vi "AnalogDisc_Core.vi"(8 "error in":errorcluster, 9 "SignalBufferQueue in":refnum<queue>, 10 "DWFCtrlQueue in":refnum<queue>, 11 "DevSN":string="210244449465") -> (0 "error out":errorcluster)   [LabVIEW 2013, in "AnalogDiscSDKLv.lvlib"]
uses:
  <instrlib>/AnalogDiscSDKLv/AnalogDiscSDKLv.lvlib
  <instrlib>/AnalogDiscSDKLv/VIs/DWF_AnalogIn_Configurations.ctl
  <instrlib>/AnalogDiscSDKLv/VIs/DWF_AcqMode.ctl
  <instrlib>/AnalogDiscSDKLv/VIs/DWF_Filter.ctl
  <instrlib>/AnalogDiscSDKLv/VIs/DWF_TrigSrc.ctl
  <instrlib>/AnalogDiscSDKLv/VIs/DWF_TrigCond.ctl
  <instrlib>/AnalogDiscSDKLv/VIs/DWF_TrigType.ctl
  <instrlib>/AnalogDiscSDKLv/VIs/DWF_CtrlQueue.ctl
  <instrlib>/AnalogDiscSDKLv/VIs/DWF_State.ctl
  <instrlib>/AnalogDiscSDKLv/VIs/DWF_PrivateStats.ctl
  <instrlib>/AnalogDiscSDKLv/VIs/DWF_InstrumentStatus.ctl
  <instrlib>/AnalogDiscSDKLv/VIs/DWF_DwfState.ctl
  <instrlib>/AnalogDiscSDKLv/VIs/DWF_Signal.ctl
  <instrlib>/AnalogDiscSDKLv/VIs/DWF_TrigLen.ctl
  <instrlib>/AnalogDiscSDKLv/VIs/DWF_DWFERC.ctl
  <vilib>/Utility/error.llb/DialogType.ctl
  <instrlib>/AnalogDiscSDKLv/VIs/DWF_AnalogOut_ChannelConfigurations.ctl
  <instrlib>/AnalogDiscSDKLv/VIs/DWF_Function.ctl
  <instrlib>/AnalogDiscSDKLv/VIs/DWF_Node.ctl
  <vilib>/Utility/miscctls.llb/LVPositionTypeDef.ctl
  <vilib>/Analysis/1siggen.llb/Ramp Pattern by Samples.vi
  <vilib>/Utility/error.llb/Error Cluster From Error Code.vi
  <vilib>/ErrorRing/Error Ring.xnode
  <vilib>/ptbypt/NI_PtbyPt.lvlib
  <userlib>/Utility/ErrorLog_lib.lvlib
  C:/Windows/System32/dwf.dll
  <vilib>/Analysis/NI_AALBase.lvlib
panel:
  out "WaitForVoltageStablize":bool
  in  "GetInfo":bool
  out "psecPosition":dbl
  out "elements":T1[](array[typedef])
  out "sysCount_inPCTrig":i32
  out "PCTrig_counter":i32
  out "AO2_sts":T3=enum."Armed"
  out "AO1_sts":T3=enum."Armed"
  in  "fStart_AO":bool
  in  "SetFuncData_AO":bool
  in  "SetTrigSrc_AO":bool
  in  "SetEnable_AO":bool
  in  "SetConfig_AO":bool
  in  "SetStates_AO":bool
  out "waited t PCTrig":u32
  out "AI_sts":T4
  in  "TriggerPC":bool
  out "Live Stats":T5
  in  "Mode(N/T)":bool caption="Mode"
  out "Graph":sgl[][](graph)
  in  "fConfig":bool
  in  "Reset":bool
  in  "CloseAll":bool
  in  "Close":bool
  in  "Enumerate":bool
  in  "Open":bool
  in  "Quit":bool
  in  "Start":bool
  in  "ConfigAll":bool
  out "UserName":string[](array[string])
  out "SN":string[](array[string])
  out "DevName":string[](array[string])
  out "DeviceID":i32[](array[numeric])
  out "pnDevice":i32
  out "isBusy":i32[](array[numeric])
  out "DeviceVersion":i32[](array[numeric])
  in  "Configurations":T6={"Acqusition"={"Freq(Hz,SampleRate)"=10000000.0, "BufferSize"=8192, "Mode"=enum."Single", "RecordLength(s)"=0.0008192}, "Channels"=[{"Range(V)"=5.0, "Offset(V)"=0.0, "Filter"=enum."Decimate", "Enable"=TRUE}], "Trigger"={"TriggerSource"=enum."None", "Timeout(s)"=0.0, "Holdoff(s)"=1e-06, "Position/Delay(s)"=0.0}, "AnalogTrigger"={"Channel"=0, "Polarity"=enum."Rising", "Type"=enum."Pulse", "Level(V)"=0.0, "Filter"=enum."MinMax", "Hysterisis(V)"=0.0}} {"AnalogTrigger"."Channel" format="%#_6p"; "AnalogTrigger"."Hysterisis(V)" format="%#_6p"; "Acqusition"."RecordLength(s)" format="%#_6p"; "Acqusition"."Freq(Hz,SampleRate)" format="%#_6p"; "Acqusition"."BufferSize" min=1 max=16384 step=1; "Trigger"."Position/Delay(s)" format="%#_6p"; "Trigger"."Holdoff(s)" format="%#_6p"}
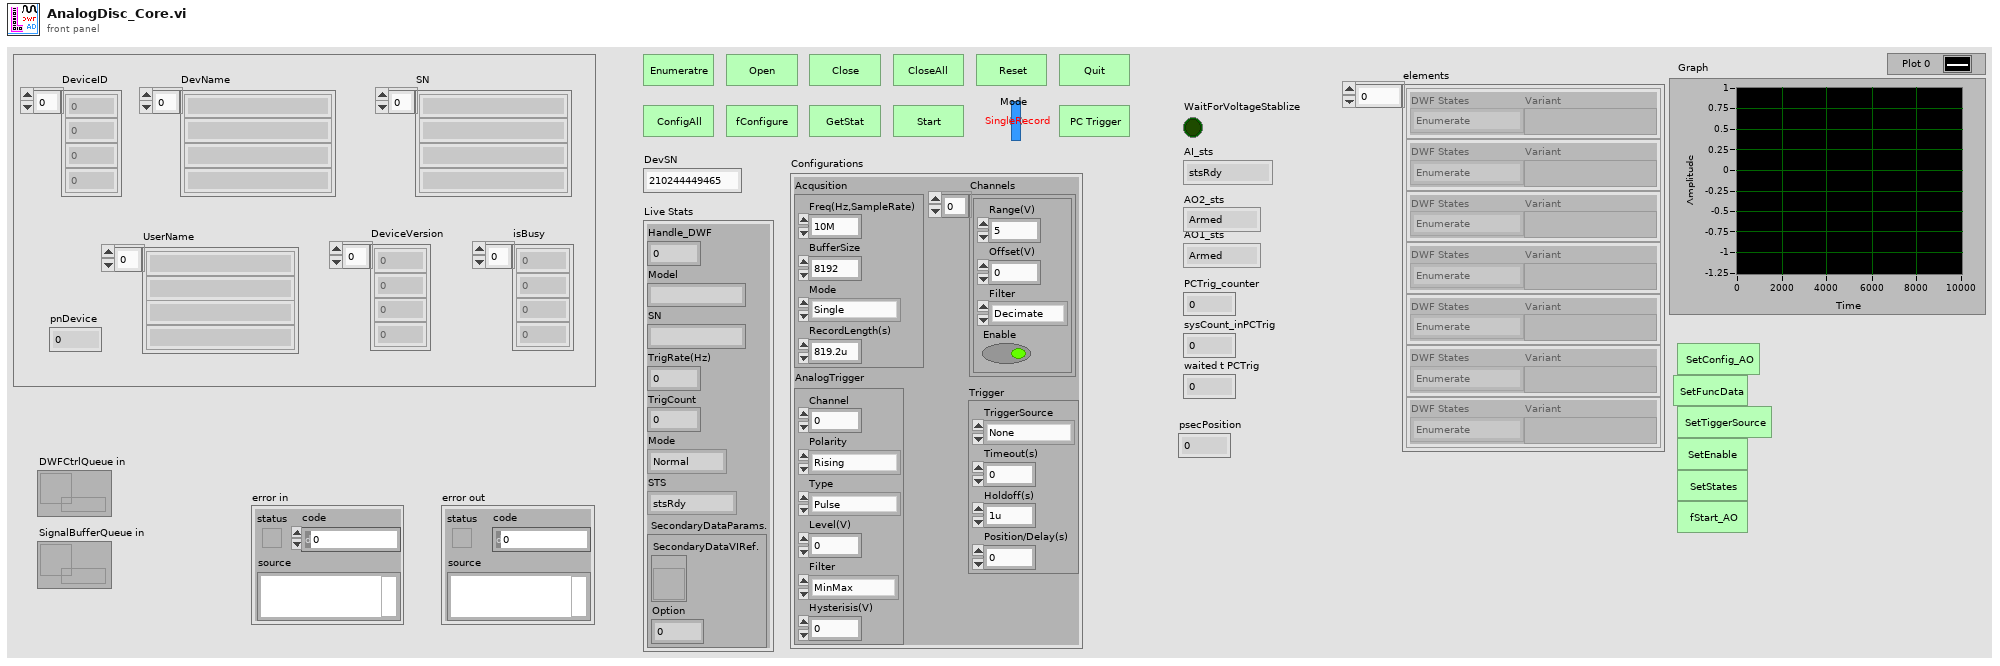
[diagram p1: front panel]
types:
  T1 = typedef "AnalogDiscSDKLv.lvlib/DWF_CtrlQueue.ctl" = cluster{"DWF States":T2, "Variant":variant}
  T2 = typedef "AnalogDiscSDKLv.lvlib/DWF_State.ctl" = enum16{"Enumerate", "Open", "Close", "CloseAll", "Reset", "Quit", "==Settings==", "SetAcquisition_", "SetChannels_", "SetTrigger_", "SetAnalogTrigDetector_", "SetAll_AcquChTrig_", "fConfigurate", "fStart", "GetStatus", "_WaitForDone/Idle", "_GetData", "GetAcquisition", "GetChannels", "GetTrigger", "GetAll_AcquChTrig", "==Messaging==", "_PushDataOut", "GetStat_", "GetConfig_", "==ModeSetup==", "SetSignalBuffer_", "SetMode_", "SetSecondaryDataRef._", "==AnalogOut==", "GetChannelCount_AO", "fStart_AO", "SetChEnable_AO", "SetConfig_AO", "SetFuncData_AO", "SetOffset_AO_", "SetMasterNode_AO", "SetStates_AO", "SetSymetry_AO", "SetTriggerSource_AO", "==Trigger==", "ManualTrigger"}
  T3 = typedef "AnalogDiscSDKLv.lvlib/DWF_DwfState.ctl" = enum16{"Ready", "Armed", "Done", "Running", "Config", "Prefill", "---", "Wait"}
  T4 = typedef "AnalogDiscSDKLv.lvlib/DWF_InstrumentStatus.ctl" = enum16{"stsRdy", "stsARM", "stsDone", "stsTrig", "stsCfg", "stsPrefill", "stsNotDone", "stsTrigDly", "stsError", "stsBusy", "stsStop"}
  T5 = typedef "AnalogDiscSDKLv.lvlib/DWF_PrivateStats.ctl" = cluster{"Handle_DWF":i32, "Model":string, "SN":string, "TrigRate(Hz)":dbl, "TrigCount":i32, "Mode":enum16{"Normal", "Turbo"}, "STS":T4, "SecondaryDataParams.":cluster{"SecondaryDataVIRef.":refnum<vi>, "Option":i32}}
  T6 = typedef "AnalogDiscSDKLv.lvlib/DWF_AnalogIn_Configurations.ctl" = cluster{"Acqusition":cluster{"Freq(Hz,SampleRate)":dbl, "BufferSize":i32, "Mode":T7, "RecordLength(s)":dbl}, "Channels":cluster{"Range(V)":dbl, "Offset(V)":dbl, "Filter":T8, "Enable":bool}[], "Trigger":cluster{"TriggerSource":T9, "Timeout(s)":dbl, "Holdoff(s)":dbl, "Position/Delay(s)":dbl}, "AnalogTrigger":cluster{"Channel":i32, "Polarity":T10, "Type":T11, "Level(V)":dbl, "Filter":T8, "Hysterisis(V)":dbl}}
  T7 = typedef "AnalogDiscSDKLv.lvlib/DWF_AcqMode.ctl" = enum16{"Single", "ScanShift", "ScanScreen", "Record"}
  T8 = typedef "AnalogDiscSDKLv.lvlib/DWF_Filter.ctl" = enum16{"Decimate", "Average", "MinMax"}
  T9 = typedef "AnalogDiscSDKLv.lvlib/DWF_TrigSrc.ctl" = enum16{"None", "PC", "DetectorAnalogIn", "DetectorDigitalIn", "AnalogIn", "DigitalIn", "DigitalOut", "AnalogOut1", "AnalogOut2", "AnalogOut3", "AnalogOut4", "External1", "External2", "External3", "External4"}
  T10 = typedef "AnalogDiscSDKLv.lvlib/DWF_TrigCond.ctl" = enum16{"Rising", "Falling"}
  T11 = typedef "AnalogDiscSDKLv.lvlib/DWF_TrigType.ctl" = enum16{"Edge", "Pulse", "Transition"}
  T12 = typedef "LVPositionTypeDef.ctl" = cluster{"Left":i32, "Top":i32}
  T13 = typedef "AnalogDiscSDKLv.lvlib/DWF_AnalogOut_ChannelConfigurations.ctl" = cluster{"FUNC":T14, "Frequency(Hz)_AO":dbl, "Amplitude(V)_AO":dbl, "Phase(deg)_AO":dbl, "Offset(V)_AO":dbl, "rgdData":dbl[], "cData":i32, "Symmetry":dbl, "Enable":bool, "Node":T15}
  T14 = typedef "AnalogDiscSDKLv.lvlib/DWF_Function.ctl" = u8
  T15 = typedef "AnalogDiscSDKLv.lvlib/DWF_Node.ctl" = enum16{"Carrier", "FM", "AM"}
  T16 = cluster{"Configs":T13[], "ChannelCount":i32, "States":cluster{"Wait(s)":dbl, "Run(s)":dbl, "cRepeat":i32, "TriggerSource":T9}[]}
  T17 = typedef "DialogType.ctl" = u16
  T18 = typedef "AnalogDiscSDKLv.lvlib/DWF_DWFERC.ctl" = enum16{"dwfercNoErc", "dwfercUnknownError", "dwfercApiLockTimeout", "dwfercAlreadyOpened", "dwfercNotSupported", "dwfercInvalidParameter0", "dwfercInvalidParameter1", "dwfercInvalidParameter2", "dwfercInvalidParameter3"}
  T19 = typedef "AnalogDiscSDKLv.lvlib/DWF_TrigLen.ctl" = enum16{"triglenLess", "triglenTimeout", "triglenMore"}
  T20 = typedef "AnalogDiscSDKLv.lvlib/DWF_Signal.ctl" = cluster{"tickcount":u32, "Signal":sgl[][], "SecondaryData":dbl[]}
  T21 = cluster{"Freq(Hz,SampleRate)":dbl, "BufferSize":i32, "Mode":T7, "RecordLength(s)":dbl}
  T22 = cluster{"Range(V)":dbl, "Offset(V)":dbl, "Filter":T8, "Enable":bool}[]
  T23 = cluster{"TriggerSource":T9, "Timeout(s)":dbl, "Holdoff(s)":dbl, "Position/Delay(s)":dbl}
  T24 = cluster{"Channel":i32, "Polarity":T10, "Type":T11, "Level(V)":dbl, "Filter":T8, "Hysterisis(V)":dbl}
  T25 = cluster{"SecondaryDataVIRef.":refnum<vi>, "Option":i32}
  T26 = cluster{"Wait(s)":dbl, "Run(s)":dbl, "cRepeat":i32, "TriggerSource":T9}[]
  T27 = cluster{"Wait(s)":dbl, "Run(s)":dbl, "cRepeat":i32, "TriggerSource":T9}
  T28 = cluster{i32, "States":cluster{"Wait(s)":dbl, "Run(s)":dbl, "cRepeat":i32, "TriggerSource":T9}}
  T29 = typedef "DWF_AnalogIn_Configurations.ctl" = cluster{"Acqusition":cluster{"Freq(Hz,SampleRate)":dbl, "BufferSize":i32, "Mode":T30, "RecordLength(s)":dbl}, "Channels":cluster{"Range(V)":dbl, "Offset(V)":dbl, "Filter":T31, "Enable":bool}[], "Trigger":cluster{"TriggerSource":T32, "Timeout(s)":dbl, "Holdoff(s)":dbl, "Position/Delay(s)":dbl}, "AnalogTrigger":cluster{"Channel":i32, "Polarity":T33, "Type":T34, "Level(V)":dbl, "Filter":T31, "Hysterisis(V)":dbl}}
  T30 = typedef "DWF_AcqMode.ctl" = enum16{"Single", "ScanShift", "ScanScreen", "Record"}
  T31 = typedef "DWF_Filter.ctl" = enum16{"Decimate", "Average", "MinMax"}
  T32 = typedef "DWF_TrigSrc.ctl" = enum16{"None", "PC", "DetectorAnalogIn", "DetectorDigitalIn", "AnalogIn", "DigitalIn", "DigitalOut", "AnalogOut1", "AnalogOut2", "AnalogOut3", "AnalogOut4", "External1", "External2", "External3", "External4"}
  T33 = typedef "DWF_TrigCond.ctl" = enum16{"Rising", "Falling"}
  T34 = typedef "DWF_TrigType.ctl" = enum16{"Edge", "Pulse", "Transition"}
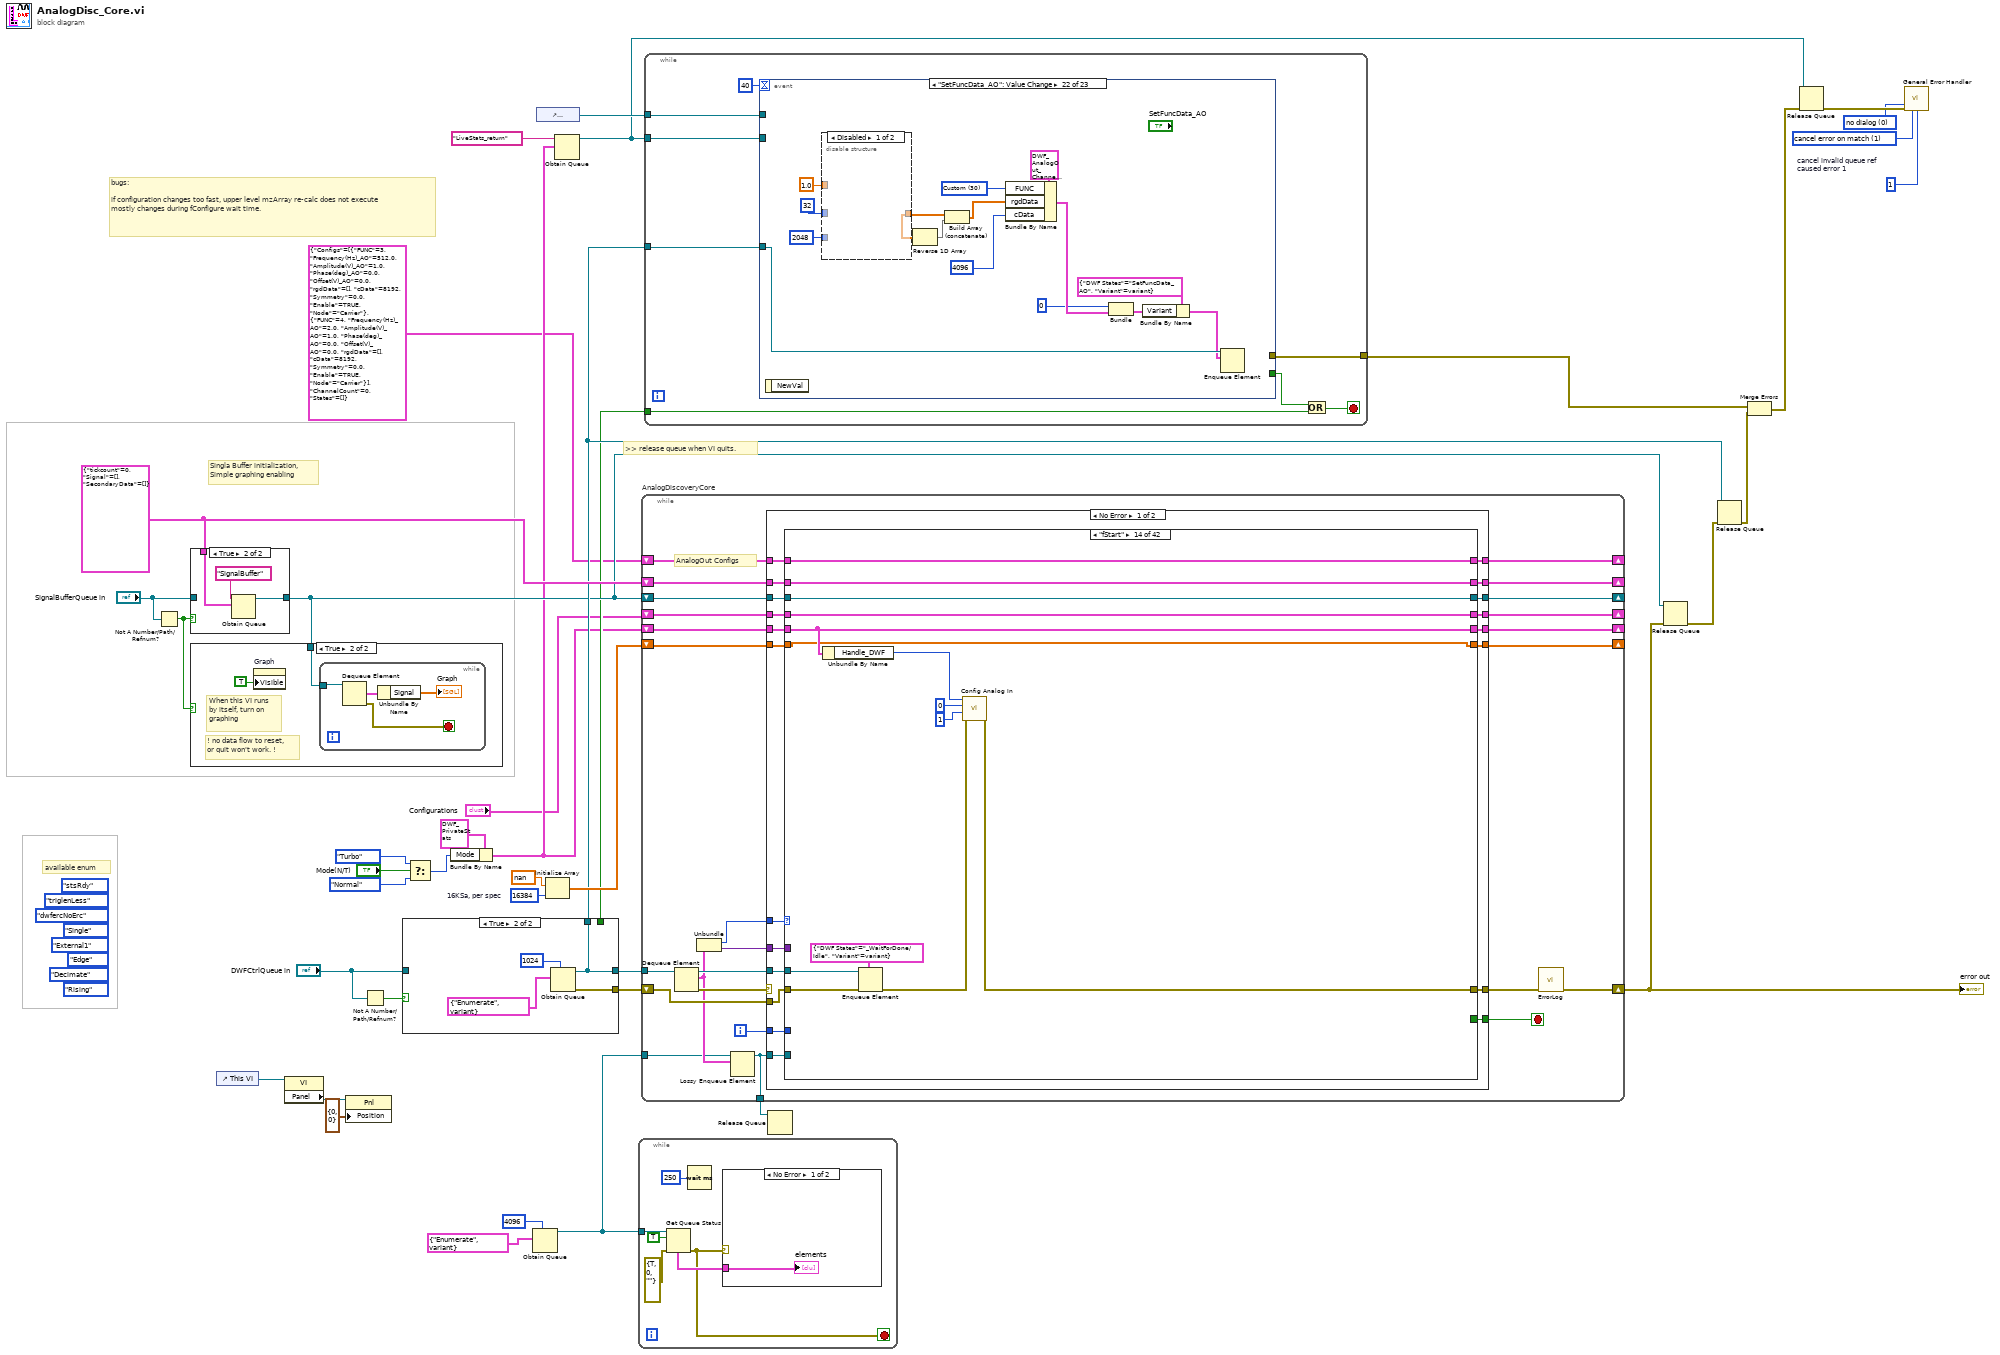
[diagram p0: block diagram]
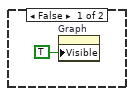
[diagram p3: hidden frame]
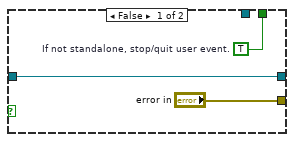
[diagram p5: hidden frame]
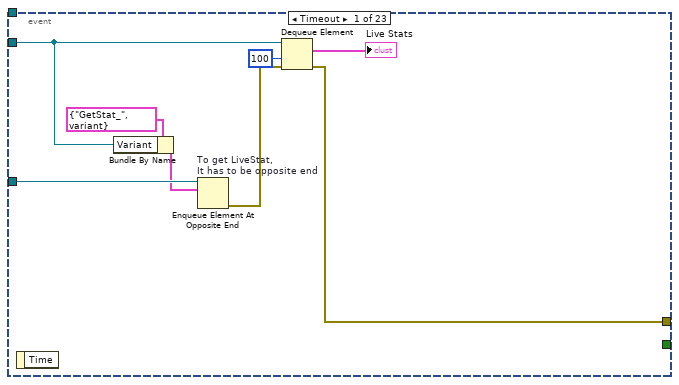
[diagram p6: hidden frame]
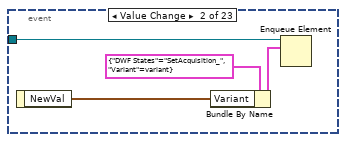
[diagram p7: hidden frame]
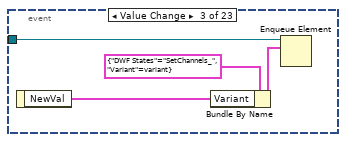
[diagram p8: hidden frame]
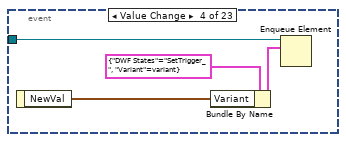
[diagram p9: hidden frame]
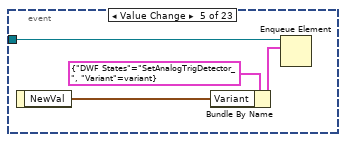
[diagram p10: hidden frame]
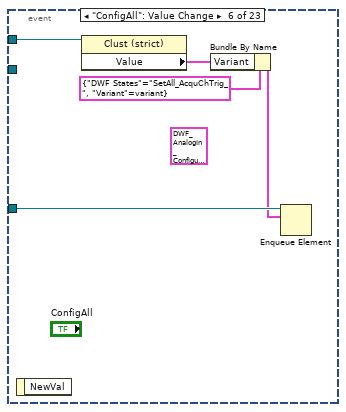
[diagram p11: hidden frame]
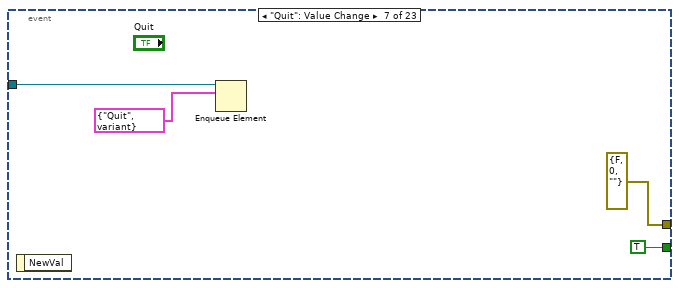
[diagram p12: hidden frame]
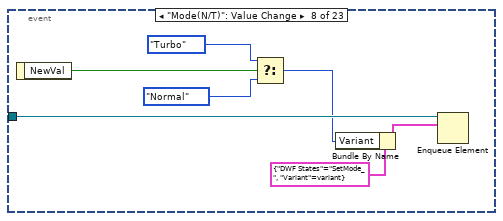
[diagram p13: hidden frame]
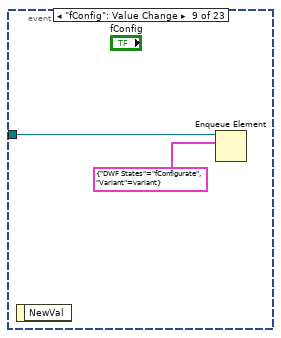
[diagram p14: hidden frame]
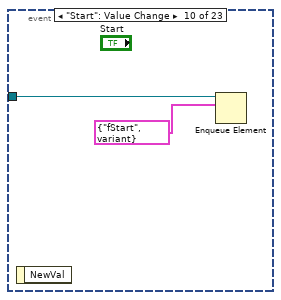
[diagram p15: hidden frame]
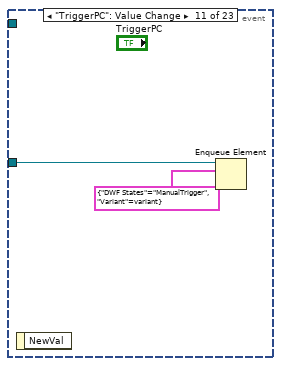
[diagram p16: hidden frame]
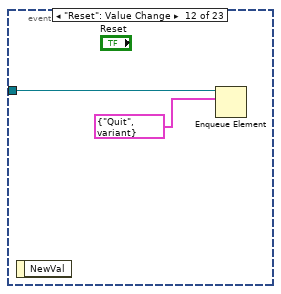
[diagram p17: hidden frame]
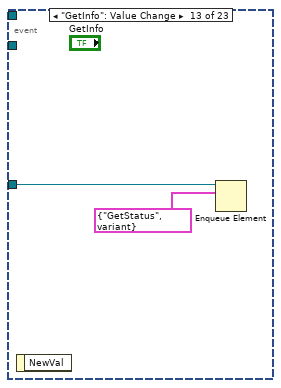
[diagram p18: hidden frame]
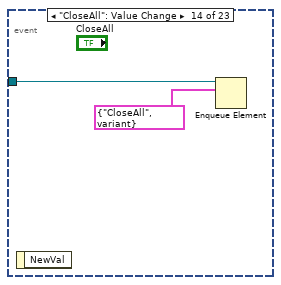
[diagram p19: hidden frame]
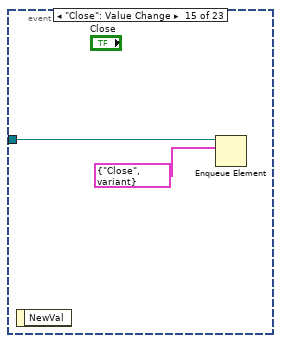
[diagram p20: hidden frame]
diagram:
  w19 = 1  # cancel invalid queue ref caused error 1
  w20 = 1 items=["no exception", "cancel error on match", "set error on match"] ("[exception action] (none:0)")
  w21 = T17 0 items=["no dialog", "OK message", "continue or stop message", "OK message + warnings", "continue/stop + warnings"] ("type of dialog (OK msg:1)")
  (unwired) DWF_TrigSrc."External1" ("TriggerSource")
  (unwired) DWF_DWFERC."dwfercNoErc" ("DWFErC")
  (unwired) DWF_TrigLen."triglenLess" ("TrigLen")
  (unwired) DWF_TrigCond."Rising" ("TrigCond")
  (unwired) DWF_TrigType."Edge" ("TrigType")
  (unwired) DWF_Filter."Decimate" ("Filter")
  (unwired) DWF_AcqMode."Single" ("ACQMODE")
  (unwired) DWF_InstrumentStatus."stsRdy" ("STS")
  w38 = 16384  # 16KSa, per spec
  w40 = T20 {"tickcount"=0, "Signal"=[], "SecondaryData"=[]} ("Signal_Typedef")
  # "bugs:\n\nif configuration changes too fast, upper level mzArray re-calc does not execute\nmostly changes during fConfigure wait time."
  # "Singla Buffer initialization,\nSimple graphing enabling"
  # "available enum"
  # ">> release queue when VI quits."
  n1 = Not A Number/Path/Refnum?(number/path/refnum="SignalBufferQueue in") -> (NaN/Path/Refnum?=w24:bool)
  n2 = case shown="True" w24 {
    tunnel: w40 -> [_ w44]
    tunnel: [w41 w43] -> w25
    tunnel: "SignalBufferQueue in" -> [w41 _]
    frame False {
    }
    frame True {
      n3 = Obtain Queue(name (unnamed)="SignalBuffer", element data type=w44) -> (queue out=w43:refnum<queue>)  [unwired: 3 in, 2 out]
    }
  }
  n4 = case shown="True" w24 {
    tunnel: w25 -> [_ w47]
    frame False {
      n5 = property on="Graph" class="WFGraph (strict)"("Visible"=TRUE) -> ()  [unwired: 2 in, 2 out]
    }
    frame True {
      # "! no data flow to reset,\nor quit won't work. !"
      # "When this VI runs\nby itself, turn on \ngraphing"
      n6 = property on="Graph" class="WFGraph (strict)"("Visible"=TRUE) -> ()  [unwired: 2 in, 2 out]
      n7 = while {
        tunnel: w47 -> [w51]
        stop <- w48 stop-if-true
        n8 = Dequeue Element(queue=w51) -> (element=w50:T20, error out=w48:errorcluster)  [unwired: 2 in, 2 out]
        n9 = Unbundle By Name(w50) -> ("Signal"=→"Graph":sgl[][])
      }
    }
  }
  n10 = control-ref of="This VI"() -> (w3:refnum<vi>)
  n11 = property class="VI"(reference=w3) -> ("Panel"=w2:refnum<vi>)  [unwired: 1 in, 2 out]
  n12 = property class="Pnl"(reference=w2, "Position"=T12 {"Left"=0, "Top"=0}) -> ()  [unwired: 1 in, 2 out]
  n13 = Not A Number/Path/Refnum?(number/path/refnum="DWFCtrlQueue in") -> (NaN/Path/Refnum?=w34:bool)
  n14 = case shown="True" w34 {
    tunnel: [w54 w55] -> w36
    tunnel: ["error in" w58] -> w35
    tunnel: "DWFCtrlQueue in" -> [w54 _]
    tunnel: [_ w55] -> w30
    tunnel: [w52 _] -> w18
    frame False {
      w52 = TRUE  # If not standalone, stop/quit user event.
    }
    frame True {
      n15 = Obtain Queue(max queue size (-1, unlimited)=1024, element data type=T1 {"DWF States"=enum."Enumerate", "Variant"=variant}) -> (queue out=w55:refnum<queue>, error out=w58:errorcluster)  [unwired: 3 in, 1 out]
    }
  }
  n16 = Select(t=enum16{"Normal", "Turbo"}."Turbo" ("Mode"), s="Mode(N/T)", f=enum16{"Normal", "Turbo"}."Normal" ("Mode")) -> (s? t:f=w11:enum16{"Normal", "Turbo"})
  n17 = Bundle By Name(cluster=T5 {"Handle_DWF"=0, "Model"="", "SN"="", "TrigRate(Hz)"=0.0, "TrigCount"=0, "Mode"=enum."Normal", "STS"=enum."stsRdy", "SecondaryDataParams."={"SecondaryDataVIRef."=refnum, "Option"=0}} ("PrivateStats(Live)"), "Mode"=w11) -> (w15:T5)
  n18 = Obtain Queue(max queue size (-1, unlimited)=4096, element data type=T1 {"DWF States"=enum."Enumerate", "Variant"=variant}) -> (queue out=w5:refnum<queue>)  [unwired: 3 in, 2 out]
  n19 = control-ref of="Configurations"() -> (w32:refnum<vi>)
  n20 = Initialize Array(nan ("Numeric"), w38) -> (w37:dbl[])
  n21 = Obtain Queue(name (unnamed)="LiveStats_return", element data type=w15) -> (queue out=w28:refnum<queue>)  [unwired: 3 in, 2 out]
  n22 = while {
    tunnel: w5 -> [w64]
    stop <- w61 stop-if-true
    n23 = Get Queue Status(queue=w64, return elements? (F)=TRUE, error in (no error)=errorcluster {"status"=TRUE, "code"=0, "source"=""}) -> (error out=w61:errorcluster, elements=w62:T1[])  [unwired: 6 out]
    n24 = Wait (ms)(milliseconds to wait=u32 250) -> ()  [unwired: 1 out]
    n25 = case shown="No Error" w61 {
      tunnel: w62 -> [w65 _]
      frame No Error {
        "elements" <- w65
      }
      frame Error {
      }
    }
  }
  n26 = while "AnalogDiscoveryCore" {
    shift-right: [w89] -> _
    shift-left: w25 -> [w90]
    tunnel: w36 -> [w71]
    shift-right: [w70] -> w23
    shift-left: w35 -> [w77]
    shift-right: [w86] -> _
    shift-left: "Configurations" -> [w85]
    shift-right: [w78] -> _
    shift-left: w15 -> [w84]
    shift-right: [w79] -> _
    shift-left: w37 -> [w82]
    shift-right: [w80] -> _
    shift-left: w40 -> [w83]
    shift-right: [w73] -> _
    shift-left: T16 {"Configs"=[{"FUNC"=3, "Frequency(Hz)_AO"=512.0, "Amplitude(V)_AO"=1.0, "Phase(deg)_AO"=0.0, "Offset(V)_AO"=0.0, "rgdData"=[], "cData"=8192, "Symmetry"=0.0, "Enable"=TRUE, "Node"=enum."Carrier"}, {"FUNC"=4, "Frequency(Hz)_AO"=2.0, "Amplitude(V)_AO"=1.0, "Phase(deg)_AO"=0.0, "Offset(V)_AO"=0.0, "rgdData"=[], "cData"=8192, "Symmetry"=0.0, "Enable"=TRUE, "Node"=enum."Carrier"}], "ChannelCount"=0, "States"=[]} -> [w74]
    tunnel: w5 -> [w68]
    tunnel: [w66] -> w4
    i -> [w72]
    stop <- w88 stop-if-true
    # "AnalogOut Configs"
    n27 = Dequeue Element(queue=w71) -> (queue out=w75:refnum<queue>, element=w69:T1, error out=w76:errorcluster)  [unwired: 2 in, 1 out]
    n28 = Unbundle(w69) -> ("DWF States"=w67:T2, "Variant"=w81:variant)
    n29 = Lossy Enqueue Element(queue=w68, element=w69) -> (queue out=w66:refnum<queue>)  [unwired: 1 in, 3 out]
    n30 = case shown="No Error" w76 {
      tunnel: w90 -> [w110 w1240]
      tunnel: [w109 w1240] -> w89
      tunnel: [w108 TRUE] -> w88
      tunnel: [w107 w1238] -> w87
      tunnel: [w106 w1241] -> w86
      tunnel: w85 -> [w105 w1241]
      tunnel: w84 -> [w104 w1242]
      tunnel: w83 -> [w103 w1239]
      tunnel: w82 -> [w102 w1243]
      tunnel: w75 -> [w101 _]
      tunnel: w67 -> [w100 _]
      tunnel: w81 -> [w99 _]
      tunnel: [w98 w1239] -> w80
      tunnel: [w97 w1243] -> w79
      tunnel: [w96 w1242] -> w78
      tunnel: w77 -> [w95 _]
      tunnel: w74 -> [w94 w1237]
      tunnel: [w93 w1237] -> w73
      tunnel: w72 -> [w92 _]
      tunnel: w66 -> [w91 _]
      frame No Error {
        n31 = case shown="\"fStart\"" w100 {
          tunnel: w110 -> [w125 w138 w219 w227 w243 w259 w283 w302 w336 w372 w402 w431 w475 w491 w504 w528 w594 w621 w628 w635 w647 w659 w666 w710 w722 w734 w743 w778 w802 w809 w820 w835 w863 w907 w968 w1013 w1055 w1104 w1152 w1188 w1195 w1216]
          tunnel: [w125 w138 w219 w227 w243 w259 w283 w302 w336 w372 w402 w431 w475 w491 w504 w528 w594 w621 w628 w635 w647 w659 w666 w710 w722 w734 w743 w779 w802 w809 w820 w835 w863 w907 w968 w1013 w1055 w1104 w1152 w1188 w1195 w1216] -> w109
          tunnel: [_ _ _ _ _ w253 _ _ _ _ _ _ _ _ _ _ _ _ _ _ _ _ _ _ _ _ _ _ _ _ _ _ _ _ _ _ _ _ _ _ _ _] -> w108
          tunnel: w101 -> [_ _ _ _ w239 w250 _ _ _ _ _ w427 _ w478 _ w530 w582 _ _ _ _ _ w682 _ _ _ _ _ _ _ _ _ _ _ _ _ _ _ _ _ _ _]
          tunnel: w95 -> [w116 w132 w211 w226 w238 w251 _ w293 w327 w364 w395 w421 w468 w482 w498 w529 w580 w620 w627 w634 w637 _ w684 w704 w712 _ w748 w775 w791 w808 w810 w822 w853 w898 w959 w1004 w1046 w1095 w1137 w1182 _ w1209]
          tunnel: [w117 w129 w210 w226 w237 w252 w278 w294 w328 w361 w392 w426 w462 w484 w497 w522 w584 w620 w627 w634 w638 w654 w683 w703 w713 w729 w744 w776 w792 w808 w811 w823 w854 w899 w960 w1005 w1047 w1096 w1144 w1177 w1189 w1210] -> w107
          tunnel: [w124 w137 w218 w225 w242 w258 w282 w299 w333 w369 w399 w424 w474 w490 w503 w527 w599 w619 w626 w633 w639 w658 w686 w702 w714 w733 w752 w784 w801 w807 w819 w834 w862 w906 w967 w1012 w1054 w1103 w1151 w1187 w1194 w1215] -> w106
          tunnel: w105 -> [w124 w137 w218 w225 w242 w258 w282 w297 w331 w367 w397 w424 w474 w490 w503 w527 w599 w619 w626 w633 w639 w658 w686 w702 w714 w733 w752 w784 w801 w807 w819 w834 w862 w906 w967 w1012 w1054 w1103 w1151 w1187 w1194 w1215]
          tunnel: [w123 w135 w214 w224 w236 w255 w281 w300 w334 w370 w400 w430 w470 w486 w496 w519 w577 w618 w625 w632 w646 w657 w680 w701 w721 w732 w745 w783 w798 w806 w815 w831 w859 w903 w964 w1009 w1051 w1100 w1148 w1184 w1193 w1211] -> w96
          tunnel: w104 -> [w123 w134 w215 w224 w236 w255 w281 w300 w334 w370 w400 w430 w470 w486 w500 w520 w587 w618 w625 w632 w646 w657 w670 w701 w721 w732 w742 w783 w797 w806 w815 w831 w859 w903 w964 w1009 w1051 w1100 w1148 w1184 w1193 w1211]
          tunnel: w103 -> [w122 w136 w217 w223 w241 w257 w280 w301 w335 w371 w401 w429 w473 w489 w502 w525 w593 w617 w624 w631 w645 w656 w679 w709 w720 w731 w751 w782 w800 w805 w818 w833 w861 w905 w966 w1011 w1053 w1102 w1150 w1186 w1192 w1214]
          tunnel: w102 -> [w115 w133 w212 w222 w240 w256 w279 w290 w325 w362 w393 w428 w467 w480 w501 w521 w598 w616 w623 w630 w644 w655 w681 w708 w719 w730 w750 w781 w799 w804 w817 w832 w860 w904 w965 w1010 w1052 w1101 w1149 w1185 w1191 w1213]
          tunnel: w99 -> [_ w131 _ _ _ _ _ w298 w332 w368 w398 w425 _ _ _ _ _ _ _ _ w643 _ _ w705 w718 _ w749 w780 w796 _ _ w829 w857 w901 w962 w1007 w1049 w1098 w1146 w1183 _ _]
          tunnel: [w122 w136 w217 w223 w241 w257 w280 w301 w335 w371 w401 w429 w473 w489 w502 w525 w592 w617 w624 w631 w645 w656 w679 w709 w720 w731 w751 w782 w800 w805 w818 w833 w861 w905 w966 w1011 w1053 w1102 w1150 w1186 w1192 w1214] -> w98
          tunnel: [w115 w133 w212 w222 w240 w256 w279 w291 w325 w362 w393 w428 w467 w480 w501 w521 w578 w616 w623 w630 w644 w655 w681 w708 w719 w730 w750 w781 w799 w804 w817 w832 w860 w904 w965 w1010 w1052 w1101 w1149 w1185 w1191 w1213] -> w97
          tunnel: w94 -> [w111 w126 w209 w220 w230 w248 w277 w289 w324 w360 w391 w420 w466 w479 w494 w506 w574 w615 w622 w629 w636 w653 w669 w699 w711 w728 w740 w772 w790 w803 w816 w828 w851 w892 w953 w998 w1040 w1091 w1140 w1176 w1190 w1212]
          tunnel: [w111 w126 w209 w220 w230 w248 w277 w289 w324 w360 w391 w420 w466 w479 w494 w506 w574 w615 w622 w629 w636 w653 w669 w699 w711 w728 w740 w772 w790 w803 w813 w828 w850 w891 w952 w997 w1039 w1090 w1139 w1176 w1190 w1212] -> w93
          tunnel: w92 -> [_ _ _ _ _ _ _ _ _ _ _ _ _ _ _ _ _ _ _ _ _ _ _ _ _ _ _ _ _ _ _ _ _ _ _ _ _ _ _ _ _ w1201]
          tunnel: w91 -> [_ _ _ _ _ _ _ _ _ _ _ _ _ _ _ _ _ _ _ _ _ _ _ _ _ _ _ _ _ _ _ _ _ _ _ _ _ _ _ _ _ _]
          frame "Enumerate" {
            n32 = call <instrlib>:"Enum Dev.vi"("error in (no error)"=w116) -> ("DeviceVersion"=→"DeviceVersion":i32[], "isBusy"=→"isBusy":i32[], "pnDevice"=→"pnDevice":i32, "DevName"=→"DevName":string[], "SN"=→"SN":string[], "UserName"=→"UserName":string[], "DeviceID"=→"DeviceID":i32[], "error out"=w117:errorcluster)  [unwired: 7 in]
          }
          frame "Open" {
            n33 = Variant To Data(error in=w132, type="", Variant=w131) -> (data=w128:string, error out=w127:errorcluster)
            n34 = case shown="Error" w127 {
              tunnel: [w147 w191] -> w135
              tunnel: w134 -> [w146 w190]
              tunnel: [w144 w189] -> w129
              tunnel: w128 -> [w142 _]
              frame No Error {
                n35 = call <instrlib>:"Enum Dev.vi"() -> ("DevName"=w141:string[], "SN"=w145:string[], "error out"=w143:errorcluster)  [unwired: 8 in, 5 out]
                n36 = Search 1D Array "find index of the dev by SN"(1D array=w145, element=w142) -> (index of element=w139:i32)  [unwired: 1 in]
                n37 = Less Than 0?(x=w139) -> (x < 0?=w140:bool)
                n38 = case shown="False" w140 {
                  tunnel: [w157 w175] -> w147
                  tunnel: w146 -> [w156 w175]
                  tunnel: [w153 w176] -> w144
                  tunnel: w143 -> [w151 _]
                  tunnel: w142 -> [w150 _]
                  tunnel: w141 -> [w149 _]
                  tunnel: w139 -> [w148 _]
                  frame False {
                    # "<<= null  to -1,\nwhich mean the first\navailable device."
                    n39 = call <vilib>:"Clear Errors.vi"("error in (no error)"=w151) -> ("error out"=w154:errorcluster)  [unwired: 6 in]
                    n40 = call <instrlib>:"Open Dev.vi"("error in (no error)"=w154, "idxDev"=w148) -> ("error out"=w155:errorcluster, "hdwf"=w152:i32)  [unwired: 7 in, 1 out]
                    n41 = case shown="Error" w155 {
                      selector: w155 -> [w161 _]
                      tunnel: [w167 w169] -> w157
                      tunnel: w152 -> [w164 _]
                      tunnel: w156 -> [w163 w169]
                      tunnel: w150 -> [w162 _]
                      tunnel: [w161 w168] -> w153
                      tunnel: w149 -> [w160 _]
                      tunnel: w148 -> [w158 _]
                      frame No Error {
                        n42 = Index Array(array=w160, index=w158) -> (element=w159:string)
                        n43 = Bundle By Name(cluster=w163, "Handle_DWF"=w164, "SN"=w162, "TrigRate(Hz)"=0.0, "TrigCount"=0, "Model"=w159) -> (w167:T5)
                      }
                      frame Error {
                        n44 = xnode "Error Ring"() -> ("error out"=w168:errorcluster)
                      }
                    }
                  }
                  frame True {
                    n45 = xnode "Error Ring"() -> ("error out"=w176:errorcluster)
                  }
                }
              }
              frame Error {
                w184 = -1  # open first avaiable device
                n46 = call <instrlib>:"Enum Dev.vi"() -> ("DevName"=w187:string[], "SN"=w183:string[], "error out"=w188:errorcluster)  [unwired: 8 in, 5 out]
                n47 = call <vilib>:"Clear Errors.vi"("error in (no error)"=w188) -> ("error out"=w185:errorcluster)  [unwired: 6 in]
                n48 = call <instrlib>:"Open Dev.vi"("error in (no error)"=w185, "idxDev"=w184) -> ("error out"=w186:errorcluster, "hdwf"=w182:i32)  [unwired: 7 in, 1 out]
                n49 = case shown="Error" w186 {
                  selector: w186 -> [w197 _]
                  tunnel: [w201 w203] -> w191
                  tunnel: w190 -> [w198 w203]
                  tunnel: [w197 w202] -> w189
                  tunnel: w187 -> [w196 _]
                  tunnel: w183 -> [w194 _]
                  tunnel: w182 -> [w192 _]
                  frame No Error {
                    n50 = Index Array(array=w196) -> (element=w195:string)  [unwired: 1 in]
                    n51 = Index Array(array=w194) -> (element=w193:string)  [unwired: 1 in]
                    n52 = Bundle By Name(cluster=w198, "TrigRate(Hz)"=0.0, "TrigCount"=0, "Model"=w195, "SN"=w193, "Handle_DWF"=w192) -> (w201:T5)
                  }
                  frame Error {
                    n53 = xnode "Error Ring"() -> ("error out"=w202:errorcluster)
                  }
                }
              }
            }
          }
          frame "Close" {
            n54 = Unbundle By Name(w215) -> ("Handle_DWF"=w216:i32)
            n55 = call <instrlib>:"Close Dev.vi"("error in (no error)"=w211, "hdwf"=w216) -> ("error out"=w210:errorcluster)  [unwired: 8 in, 1 out]
            n56 = Bundle By Name(cluster=w215, "Handle_DWF"=-1) -> (w214:T5)
          }
          frame "CloseAll" {
            n57 = for {
              N: 4 -> [_]
              i -> [w229]
              n58 = call <instrlib>:"Close Dev.vi"("hdwf"=w229) -> ("error out"=w228:errorcluster)  [unwired: 9 in, 1 out]
              n59 = call <vilib>:"Clear Errors.vi"("error in (no error)"=w228) -> ()  [unwired: 6 in, 1 out]
            }
          }
          frame "Reset" {
            n60 = Unbundle By Name(w236) -> ("SN"=w234:string)
            n61 = Bundle By Name(cluster=T1 {"DWF States"=enum."Open", "Variant"=variant} ("element"), "Variant"=w234) -> (w233:T1)
            n62 = Build Array(w233, T1 {"DWF States"=enum."Close", "Variant"=variant} ("element")) -> (w231:T1[])
            n63 = for {
              tunnel: w239 -> [w247]
              tunnel: w231 -> [w244] mode=indexing
              shift-right: [w245] -> w237
              shift-left: w238 -> [w246]
              n64 = Enqueue Element At Opposite End(queue=w247, element=w244, error in (no error)=w246) -> (error out=w245:errorcluster)  [unwired: 1 in, 2 out]
            }
          }
          frame "Quit" {
            n65 = Unbundle By Name(w255) -> ("SecondaryDataParams..SecondaryDataVIRef."=w249:refnum<vi>, "Handle_DWF"=w254:i32)
            n66 = case "Check handle leak??" shown="-1" w254 {
              tunnel: [_ TRUE] -> w253
              tunnel: [w261 w270] -> w252
              tunnel: w251 -> [w262 w271]
              tunnel: w250 -> [w263 _]
              tunnel: w249 -> [_ w268]
              frame Default {
                n67 = for {
                  tunnel: w263 -> [w267]
                  tunnel: T1[] [{"DWF States"=enum."Quit", "Variant"=variant}, {"DWF States"=enum."Close", "Variant"=variant}] -> [w264] mode=indexing
                  shift-right: [w265] -> w261
                  shift-left: w262 -> [w266]
                  n68 = Enqueue Element At Opposite End(queue=w267, element=w264, error in (no error)=w266) -> (error out=w265:errorcluster)  [unwired: 1 in, 2 out]
                }
              }
              frame -1 {
                n69 = Not A Number/Path/Refnum?(number/path/refnum=w268) -> (NaN/Path/Refnum?=w269:bool)
                n70 = case shown="False" w269 {
                  tunnel: w268 -> [w275 _]
                  tunnel: w271 -> [w274 w276]
                  tunnel: [w273 w276] -> w270
                  frame False {
                    n71 = Close Reference "Release secondarydatavi Reference"(reference=w275, error in (no error)=w274) -> (error out=w273:errorcluster)
                  }
                  frame True {
                  }
                }
              }
            }
          }
          frame "==Settings==" {
            # "Invalid frame"
            n72 = xnode "Error Ring"() -> ("error out"=w278:errorcluster)
          }
          frame "SetAcquisition_" {
            n73 = Unbundle By Name(w297) -> ("Acqusition"=w296:T21)
            n74 = Variant To Data(error in=w293, type=w296, Variant=w298) -> (data=w295:T21, error out=w292:errorcluster)
            n75 = Bundle By Name(cluster=w297, "Acqusition"=w295) -> (w299:T6)
            n76 = case shown="No Error" w292 {
              selector: w292 -> [w309 _]
              tunnel: w300 -> [w316 _]
              tunnel: w295 -> [w314 _]
              tunnel: [w311 w318] -> w294
              tunnel: [w308 w317] -> w291
              tunnel: w290 -> [_ w317]
              frame No Error {
                n77 = Unbundle By Name(w314) -> ("Mode"=w313:T7, "Freq(Hz,SampleRate)"=w312:dbl, "BufferSize"=w306:i32, "RecordLength(s)"=w303:dbl)
                n78 = Unbundle By Name(w316) -> ("Handle_DWF"=w315:i32)
                n79 = call <instrlib>:"Set Acquisition Config Analog In.vi"("RecordLength(s)"=w303, "AcqMode"=w313, "error in (no error)"=w309, "BufferSize"=w306, "Frquency(MS/s)"=w312, "hdwf"=w315) -> ("error out"=w311:errorcluster)  [unwired: 3 in, 2 out]
                n80 = In Range and Coerce(upper limit=16384, x=w306, lower limit=1) -> (coerced(x)=w307:i32)  [unwired: 1 out]
                n81 = Initialize Array(nan ("Numeric"), w307) -> (w308:dbl[])
              }
              frame Error {
                n82 = xnode "Error Ring"() -> ("error out"=w318:errorcluster)
              }
            }
          }
          frame "SetChannels_" {
            n83 = Unbundle By Name(w331) -> ("Channels"=w330:T22)
            n84 = Variant To Data(error in=w327, type=w330, Variant=w332) -> (data=w329:T22, error out=w326:errorcluster)
            n85 = Bundle By Name(cluster=w331, "Channels"=w329) -> (w333:T6)
            n86 = case shown="No Error" w326 {
              selector: w326 -> [w337 _]
              tunnel: w334 -> [w341 _]
              tunnel: w329 -> [w339 _]
              tunnel: [w338 w352] -> w328
              frame No Error {
                n87 = Unbundle By Name(w341) -> ("Handle_DWF"=w340:i32)
                n88 = for {
                  tunnel: w340 -> [w351]
                  tunnel: w339 -> [w350] mode=indexing
                  shift-right: [w343] -> w338
                  shift-left: w337 -> [w342]
                  i -> [w344]
                  n89 = Unbundle By Name(w350) -> ("Offset(V)"=w348:dbl, "Range(V)"=w349:dbl, "Enable"=w346:bool, "Filter"=w347:T8)
                  n90 = Boolean To (0,1)(Boolean=w346) -> (0, 1=w345:i16)
                  n91 = call <instrlib>:"Set Channels Config Analog In.vi"("voltOffset"=w348, "Filter"=w347, "voltsRange"=w349, "error in (no error)"=w342, "Enable"=w345, "indexCh"=w344, "hdwf"=w351) -> ("error out"=w343:errorcluster)  [unwired: 2 in, 2 out]
                }
              }
              frame Error {
                n92 = xnode "Error Ring"() -> ("error out"=w352:errorcluster)
              }
            }
          }
          frame "SetTrigger_" {
            n93 = Unbundle By Name(w367) -> ("Trigger"=w366:T23)
            n94 = Variant To Data(error in=w364, type=w366, Variant=w368) -> (data=w365:T23, error out=w363:errorcluster)
            n95 = Bundle By Name(cluster=w367, "Trigger"=w365) -> (w369:T6)
            n96 = case shown="No Error" w363 {
              selector: w363 -> [w381 _]
              tunnel: w370 -> [w383 _]
              tunnel: w365 -> [w382 _]
              tunnel: [w377 w384] -> w361
              tunnel: [w376 _] -> w359
              tunnel: [w375 _] -> w358
              frame No Error {
                n97 = Unbundle By Name(w382) -> ("Timeout(s)"=w380:dbl, "TriggerSource"=w378:T9, "Position/Delay(s)"=w375:dbl, "Holdoff(s)"=w379:dbl)
                n98 = Unbundle By Name(w383) -> ("Handle_DWF"=w376:i32)
                n99 = call <instrlib>:"Set Analog In Trigger.vi"("secHoldOff"=w379, "secPosition"=w375, "secTimeout"=w380, "error in (no error)"=w381, "trigsrc"=w378, "hdwf"=w376) -> ("error out"=w377:errorcluster)  [unwired: 4 in, 1 out]
              }
              frame Error {
                n100 = xnode "Error Ring"() -> ("error out"=w384:errorcluster)
              }
            }
            n101 = disable-structure shown="Disabled" {
              disable-tunnel: w359 -> [w374 _]
              disable-tunnel: w358 -> [w373 _]
              frame Disabled {
                n102 = dll-call lib="C:/Windows/System32/dwf.dll" fn="FDwfAnalogInTriggerPositionSet"("hdwf"=w374, "secPosition"=w373) -> ()  [unwired: 6 in, 2 out]
              }
              frame Enabled {
              }
            }
          }
          frame "SetAnalogTrigDetector_" {
            n103 = Unbundle By Name(w397) -> ("AnalogTrigger"=w390:T24)
            n104 = Variant To Data(error in=w395, type=w390, Variant=w398) -> (data=w396:T24, error out=w394:errorcluster)
            n105 = Bundle By Name(cluster=w397, "AnalogTrigger"=w396) -> (w399:T6)
            n106 = case shown="No Error" w394 {
              selector: w394 -> [w412 _]
              tunnel: w400 -> [w413 _]
              tunnel: w396 -> [w403 _]
              tunnel: [w411 w414] -> w392
              frame No Error {
                n107 = Unbundle By Name(w413) -> ("Handle_DWF"=w410:i32)
                n108 = Unbundle By Name(w403) -> ("Hysterisis(V)"=w409:dbl, "Level(V)"=w408:dbl, "Channel"=w407:i32, "Polarity"=w406:T10, "Type"=w405:T11, "Filter"=w404:T8)
                n109 = call <instrlib>:"Set Analog In Trigger Detector.vi"("hdwf"=w410, "voltsLevel"=w408, "HystersisvoltsLevel"=w409, "idxChannel"=w407, "trigcond"=w406, "trigtype"=w405, "error in (no error)"=w412, "filter"=w404) -> ("error out"=w411:errorcluster)  [unwired: 6 in, 1 out]
              }
              frame Error {
                n110 = xnode "Error Ring"() -> ("error out"=w414:errorcluster)
              }
            }
          }
          frame "SetAll_AcquChTrig_" {
            n111 = Variant To Data(type=w424, Variant=w425) -> (data=w422:T6, error out=w423:errorcluster)  [unwired: 1 in]
            n112 = case shown="No Error" w423 {
              tunnel: w427 -> [w449 _]
              tunnel: [w448 w454] -> w426
              tunnel: w422 -> [w447 _]
              tunnel: w421 -> [w446 _]
              frame No Error {
                n113 = Unbundle By Name(w447) -> ("Acqusition"=w444:T21, "Channels"=w442:T22, "Trigger"=w440:T23, "AnalogTrigger"=w434:T24)
                n114 = Bundle By Name(cluster=T1 {"DWF States"=enum."SetAcquisition_", "Variant"=variant} ("element"), "Variant"=w444) -> (w439:T1)
                n115 = Bundle By Name(cluster=T1 {"DWF States"=enum."SetChannels_", "Variant"=variant} ("element"), "Variant"=w442) -> (w438:T1)
                n116 = Bundle By Name(cluster=T1 {"DWF States"=enum."SetTrigger_", "Variant"=variant} ("element"), "Variant"=w440) -> (w437:T1)
                n117 = Bundle By Name(cluster=T1 {"DWF States"=enum."SetAnalogTrigDetector_", "Variant"=variant} ("element"), "Variant"=w434) -> (w433:T1)
                n118 = Build Array(w439, w438, w437, w433) -> (w436:T1[])
                n119 = Reverse 1D Array(array=w436) -> (reversed array=w432:T1[])
                n120 = for {
                  tunnel: w449 -> [w453]
                  shift-right: [w452] -> w448
                  shift-left: w446 -> [w451]
                  tunnel: w432 -> [w450] mode=indexing
                  n121 = Enqueue Element At Opposite End(queue=w453, element=w450, error in (no error)=w451) -> (error out=w452:errorcluster)  [unwired: 1 in, 2 out]
                }
              }
              frame Error {
                n122 = xnode "Error Ring"() -> ("error out"=w454:errorcluster)
              }
            }
          }
          frame "fConfigurate" {
            n123 = Unbundle By Name(w470) -> ("Handle_DWF"=w469:i32)
            n124 = call <instrlib>:"Config Analog In.vi"("error in (no error)"=w468, "fStart"=0, "fReconfigure"=1, "hdwf"=w469) -> ("error out"=w465:errorcluster)  [unwired: 5 in, 2 out]
            n125 = property on="WaitForVoltageStablize" class="Bool (strict)"(error in=w465, "Value"=TRUE ("WaitForVoltageStablize")) -> (error out=w464:errorcluster)  [unwired: 1 in, 1 out]
            n126 = flat-sequence {
              tunnel: [w476] -> w463
              tunnel: w464 -> [w476]
              frame #0 {
                # "todo:\nSend Out message: \nWaiting for offest voltage stablized."
                n127 = Wait (ms) "Wait for voltage stablize \n(According to SDK manual)"(milliseconds to wait=u32 1500) -> ()  [unwired: 1 out]
              }
            }
            n128 = property on="WaitForVoltageStablize" class="Bool (strict)"(error in=w463, "Value"=FALSE ("WaitForVoltageStablize")) -> (error out=w462:errorcluster)  [unwired: 1 in, 1 out]
          }
          frame "fStart" {
            n129 = Unbundle By Name(w486) -> ("Handle_DWF"=w485:i32)
            n130 = Enqueue Element(queue=w478, element=T1 {"DWF States"=enum."_WaitForDone/Idle", "Variant"=variant}, error in (no error)=w482) -> (error out=w481:errorcluster)  [unwired: 1 in, 2 out]
            n131 = call <instrlib>:"Config Analog In.vi"("error in (no error)"=w481, "fStart"=1, "fReconfigure"=0, "hdwf"=w485) -> ("error out"=w484:errorcluster)  [unwired: 5 in, 2 out]
          }
          frame "GetStatus" {
            n132 = Unbundle By Name(w500) -> ("Handle_DWF"=w493:i32)
            n133 = call <instrlib>:"Get Status Analog In.vi"("error in (no error)"=w498, "fReadData"=0, "hdwf"=w493) -> ("error out"=w497:errorcluster, "psts"=w495:T4)  [unwired: 5 in, 1 out]
            n134 = Bundle By Name(cluster=w500, "STS"=w495) -> (w496:T5)
            n135 = dll-call lib="C:/Windows/System32/dwf.dll" fn="FDwfAnalogInTriggerPositionGet"("hdwf"=w493) -> ("psecPosition"=→"psecPosition":dbl)  [unwired: 6 in, 2 out]
          }
          frame "_WaitForDone/Idle" {
            w514 = T2[] [enum."Close", enum."CloseAll", enum."Reset", enum."Quit", enum."GetStatus"] items=["Enumerate", "Open", "Close", "CloseAll", "Reset", "Quit", "==Settings==", "SetAcquisition_", "SetChannels_", "SetTrigger_", "SetAnalogTrigDetector_", "SetAll_AcquChTrig_", "fConfigurate", "fStart", "GetStatus", "_WaitForDone/Idle", "_GetData", "GetAcquisition", "GetChannels", "GetTrigger", "GetAll_AcquChTrig", "==Messaging==", "_PushDataOut", "GetStat_", "GetConfig_", "==ModeSetup==", "SetSignalBuffer_", "SetMode_", "SetSecondaryDataRef._", "==AnalogOut==", "GetChannelCount_AO", "fStart_AO", "SetChEnable_AO", "SetConfig_AO", "SetFuncData_AO", "SetOffset_AO_", "SetMasterNode_AO", "SetStates_AO", "SetSymetry_AO", "SetTriggerSource_AO", "==Trigger==", "ManualTrigger"]
            # "Logic:\nClose => Quit\ntimeout =>"
            n136 = Unbundle By Name(w520) -> ("SecondaryDataParams..SecondaryDataVIRef."=w508:refnum<vi>, "SecondaryDataParams..Option"=w507:i32, "Handle_DWF"=w526:i32)
            n137 = Wait Until Next ms Multiple(millisecond multiple=u32 1) -> ()  [unwired: 1 out]
            n138 = call <instrlib>:"Get Status Analog In.vi"("error in (no error)"=w529, "hdwf"=w526) -> ("error out"=w511:errorcluster, "psts"=w509:T4)  [unwired: 6 in, 1 out]
            n139 = Preview Queue Element(queue=w530, timeout in ms (-1)=0, error in (no error)=w511) -> (queue out=w524:refnum<queue>, element=w517:T1, timed out?=w515:bool, error out=w523:errorcluster)
            n140 = Bundle By Name(cluster=w520, "STS"=w509) -> (w519:T5)
            n141 = Unbundle(w517) -> ("DWF States"=w505:T2)  [unwired: 1 out]
            n142 = Search 1D Array(1D array=w514, element=w505) -> (index of element=w513:i32)  [unwired: 1 in]
            n143 = Greater Or Equal To 0?(x=w513) -> (x >= 0?=w512:bool)
            n144 = Compound Arithmetic op=AND(w512, invert w515) -> (w510:bool)
            n145 = case shown="False" w510 {
              tunnel: w524 -> [w536 _]
              tunnel: w523 -> [w535 w569]
              tunnel: [w534 w569] -> w522
              tunnel: w509 -> [w533 _]
              tunnel: w508 -> [w532 _]
              tunnel: w507 -> [w531 _]
              tunnel: w505 -> [_ _]
              frame False {
                # "queue empty OR other command"
                n146 = case shown="\"stsRdy\"" w533 {
                  tunnel: w536 -> [w537 w551 _ w563]
                  tunnel: w535 -> [w540 w549 w560 w562]
                  tunnel: [w539 w550 w560 w561] -> w534
                  tunnel: w532 -> [_ w545 _ _]
                  tunnel: w531 -> [_ w548 _ _]
                  frame "stsRdy" {
                    # "Typically, this is caused by config change\nduring acquisition. \nPush fConfig and fStart to continure  acuisition."
                    n147 = for {
                      shift-right: [w543] -> w539
                      shift-left: w540 -> [w544]
                      tunnel: T1[] [{"DWF States"=enum."fConfigurate", "Variant"=variant}, {"DWF States"=enum."fStart", "Variant"=variant}] -> [w542] mode=indexing
                      tunnel: w537 -> [w541]
                      n148 = Enqueue Element(queue=w541, element=w542, error in (no error)=w544) -> (error out=w543:errorcluster)  [unwired: 1 in, 2 out]
                    }
                  }
                  frame "stsDone" {
                    n149 = Not A Number/Path/Refnum?(number/path/refnum=w545) -> (NaN/Path/Refnum?=w546:bool)
                    n150 = case shown="True" w546 {
                      tunnel: w545 -> [w555 _]
                      tunnel: w549 -> [w554 w556]
                      tunnel: w548 -> [w553 _]
                      tunnel: [w552 w556] -> w547
                      frame False {
                        n151 = call-by-ref "Maybe this give a little bit \nbetter timing precision\nfor secondary data?"(reference=w555, error in=w554, "Index"=w553) -> (error out=w552:errorcluster)  [unwired: 10 in, 2 out]
                      }
                      frame True {
                      }
                    }
                    n152 = flat-sequence {
                      tunnel: w551 -> [w559]
                      tunnel: [w557] -> w550
                      tunnel: w547 -> [w557]
                      frame #0 {
                        n153 = Enqueue Element(queue=w559, element=T1 {"DWF States"=enum."_GetData", "Variant"=variant}) -> ()  [unwired: 2 in, 3 out]
                      }
                    }
                  }
                  frame "stsError", "stsStop" {
                  }
                  frame Default {
                    n154 = disable-structure "Driven by outter layer queue timeout" shown="Enabled" {
                      disable-tunnel: w563 -> [w567 _]
                      disable-tunnel: w562 -> [w566 w568]
                      disable-tunnel: [w565 w568] -> w561
                      frame Enabled {
                        n155 = Enqueue Element(queue=w567, element=T1 {"DWF States"=enum."_WaitForDone/Idle", "Variant"=variant}, error in (no error)=w566) -> (error out=w565:errorcluster)  [unwired: 1 in, 2 out]
                      }
                      frame Disabled {
                      }
                    }
                  }
                }
              }
              frame True {
              }
            }
          }
          frame "_GetData" {
            # "If 0 channel enabled, then this should generate\n an empty array output in queue"
            n156 = Unbundle By Name(w587) -> ("TrigCount"=w575:i32, "Handle_DWF"=w586:i32, "Mode"=w583:enum16{"Normal", "Turbo"})
            n157 = Unbundle By Name(w599) -> ("Acqusition.Freq(Hz,SampleRate)"=w573:dbl, "Acqusition.RecordLength(s)"=w572:dbl, "Acqusition.BufferSize"=w570:i32, "Channels"=w596:T22)
            n158 = Enqueue Element(queue=w582, element=T1 {"DWF States"=enum."_PushDataOut", "Variant"=variant}, error in (no error)=w580) -> (error out=w579:errorcluster)  [unwired: 1 in, 2 out]
            n159 = Tick Count (ms)() -> (millisecond timer value=w597:u32)
            n160 = Array Size(array=w596) -> (size(s)=w595:i32)
            n161 = Multiply(x=w573, y=w572) -> (x*y=w571:dbl)
            n162 = Round To Nearest(number=w571) -> ()  [unwired: 1 out]
            n163 = for {
              N: w595 -> [_]
              tunnel: [w608] -> w590 mode=indexing
              tunnel: w570 -> [w614]
              shift-right: [w608] -> w578
              shift-left: w598 -> [w612]
              tunnel: [w610] -> w591
              tunnel: w597 -> [w610]
              shift-right: [w609] -> w588
              shift-left: w579 -> [w611]
              shift-right: [w606] -> w585
              shift-left: w586 -> [w607]
              i -> [w613]
              n164 = call <instrlib>:"Get Data Analog In.vi"("BufferSize"=w614, "error in (no error)"=w611, "rgdSamples"=w612, "idxChannel"=w613, "hdwf"=w607) -> ("error out"=w609:errorcluster, "rgdSamples out"=w608:dbl[], "function return"=w606:i32)  [unwired: 4 in]
            }
            n165 = Increment(x=w575) -> (x+1=w576:i32)
            n166 = To Single Precision Float(number=w590) -> (single precision float=w589:sgl[][])
            n167 = Bundle By Name(cluster=w587, "TrigCount"=w576) -> (w577:T5)
            n168 = Bundle By Name(cluster=w593, "tickcount"=w591, "Signal"=w589) -> (w592:T20)
            n169 = case shown="\"Turbo\"" w583 {
              tunnel: w588 -> [w600 w605]
              tunnel: w585 -> [_ w604]
              tunnel: [w600 w603] -> w584
              frame "Normal", Default {
              }
              frame "Turbo" {
                n170 = call <instrlib>:"Config Analog In.vi"("error in (no error)"=w605, "fStart"=1, "fReconfigure"=0, "hdwf"=w604) -> ("error out"=w603:errorcluster)  [unwired: 5 in, 2 out]
              }
            }
          }
          frame "GetAcquisition" {
          }
          frame "GetChannels" {
          }
          frame "GetTrigger" {
          }
          frame "GetAll_AcquChTrig" {
            n171 = Variant To Data(type=refnum<queue> refnum ("queue out"), Variant=w643) -> (data=w641:refnum<queue>, error out=w640:errorcluster)  [unwired: 1 in]
            n172 = case shown="No Error" w640 {
              selector: w640 -> [_ w652]
              tunnel: w641 -> [w651 _]
              tunnel: w639 -> [w650 _]
              tunnel: [w649 w652] -> w638
              tunnel: w637 -> [w648 _]
              frame No Error {
                # "short term solution, need refine\nget real result from device"
                n173 = Enqueue Element(queue=w651, element=w650, error in (no error)=w648) -> (error out=w649:errorcluster)  [unwired: 1 in, 2 out]
              }
              frame Error {
              }
            }
          }
          frame "==Messaging==" {
            # "Invalid Frame"
            n174 = xnode "Error Ring"() -> ("error out"=w654:errorcluster)
          }
          frame "_PushDataOut" {
            n175 = Unbundle By Name(w670) -> ("SecondaryDataParams..SecondaryDataVIRef."=w667:refnum<vi>)
            n176 = Unbundle By Name(w670) -> ("Mode"=w685:enum16{"Normal", "Turbo"})
            n177 = case "Actually, does NOTHING." shown="\"Turbo\"" w685 {
              tunnel: w684 -> [w692 w698]
              tunnel: [w692 w697] -> w683
              tunnel: w682 -> [_ w696]
              frame "Normal" {
              }
              frame "Turbo" {
                # "In turbo mode, \nre-arming is done in \"_GetData\"\n\nNormal mode => no need to re-arming  daq"
                n178 = Enqueue Element(queue=w696, element=T1 {"DWF States"=enum."_WaitForDone/Idle", "Variant"=variant}, error in (no error)=w698) -> (queue out=w694:refnum<queue>, error out=w697:errorcluster)  [unwired: 1 in, 1 out]
                n179 = Enqueue Element(queue=w694, element=T1 {"DWF States"=enum."fStart", "Variant"=variant}) -> ()  [unwired: 2 in, 3 out]
              }
            }
            n180 = Not A Number/Path/Refnum?(number/path/refnum=w667) -> (NaN/Path/Refnum?=w668:bool)
            n181 = case shown="False" w668 {
              tunnel: w679 -> [w690 w691]
              tunnel: w667 -> [w689 _]
              tunnel: [w687 w691] -> w665
              frame False {
                n182 = call-by-ref "Get SecondaryData"(reference=w689) -> ("SecondaryData"=w688:dbl[])  [unwired: 12 in, 2 out]
                n183 = Bundle By Name(cluster=w690, "SecondaryData"=w688) -> (w687:T20)
              }
              frame True {
              }
            }
            n184 = Enqueue Element "Send/Push Data Out"(queue=w666, element=w665) -> ()  [unwired: 2 in, 3 out]
            n185 = Unbundle By Name(w679) -> ("tickcount"=w674:u32)
            n186 = Tick Count (ms)() -> (millisecond timer value=w678:u32)
            n187 = feedback #1(w678) -> (w677:u32)
            n188 = feedback-in #1(w674) -> ()
            n189 = Subtract(x=w674, y=w677) -> (x-y=w675:u32)
            n190 = Divide(x=1000.0, y=w675) -> (x/y=w672:dbl)
            n191 = call <vilib>:"Mean PtByPt.vi"("x"=w672, "sample length"=16) -> ("mean"=w673:dbl)  [unwired: 2 in, 1 out]
            n192 = Bundle By Name(cluster=w670, "TrigRate(Hz)"=w673) -> (w680:T5)
          }
          frame "GetStat_" {
            n193 = Variant To Data(error in=w704, type=refnum<queue> refnum ("queue out"), Variant=w705) -> (data=w707:refnum<queue>, error out=w706:errorcluster)
            n194 = Enqueue Element "Send Core Stat"(queue=w707, element=w701, error in (no error)=w706) -> (error out=w703:errorcluster)  [unwired: 1 in, 2 out]
          }
          frame "GetConfig_" {
            # "solution:\n\n1 call vi ref, vi send out typed command. => possible, idea, time consuming \n\n2 make this frame specific, bad. \n\n3 user event call and wait, then send typed command.  possible, fast?"
            n195 = Variant To Data(type=refnum<queue> refnum ("queue out"), Variant=w718) -> (data=w716:refnum<queue>, error out=w715:errorcluster)  [unwired: 1 in]
            n196 = case shown="No Error" w715 {
              selector: w715 -> [_ w727]
              tunnel: w716 -> [w726 _]
              tunnel: w714 -> [w725 _]
              tunnel: [w724 w727] -> w713
              tunnel: w712 -> [w723 _]
              frame No Error {
                # "short term solution, need refine\nget real result from device"
                n197 = Enqueue Element(queue=w726, element=w725, error in (no error)=w723) -> (error out=w724:errorcluster)  [unwired: 1 in, 2 out]
              }
              frame Error {
              }
            }
          }
          frame "==ModeSetup==" {
            # "Invalid Frame"
            n198 = xnode "Error Ring"() -> ("error out"=w729:errorcluster)
          }
          frame "SetSecondaryDataRef._" {
            n199 = Unbundle By Name(w742) -> ("SecondaryDataParams."=w741:T25)
            n200 = Variant To Data(error in=w748, type=w741, Variant=w749) -> (data=w746:T25, error out=w747:errorcluster)
            n201 = case shown="No Error" w747 {
              tunnel: w746 -> [w756 _]
              tunnel: w742 -> [w764 w766]
              tunnel: [w763 w766] -> w745
              tunnel: [_ w765] -> w744
              tunnel: w741 -> [w757 _]
              frame No Error {
                n202 = Unbundle By Name(w757) -> ("SecondaryDataVIRef."=w754:refnum<vi>)
                n203 = Unbundle By Name(w756) -> ("Option"=w753:i32, "SecondaryDataVIRef."=w755:refnum<vi>)
                n204 = property class="VI Interface Type 0"(reference=w755) -> (reference out=w760:refnum<vi>, "Path"=w762:path)  [unwired: 1 in, 1 out]
                n205 = Close Reference(reference=w754) -> (error out=w758:errorcluster)  [unwired: 1 in]
                n206 = call <vilib>:"Clear Errors.vi"("error in (no error)"=w758) -> ()  [unwired: 6 in, 1 out]
                n207 = Open VI Reference(type specifier VI Refnum (for type only)=w760, vi path=w762, options=256) -> (vi reference=w759:refnum<vi>)  [unwired: 3 in, 1 out]
                n208 = Bundle By Name(cluster=w764, "SecondaryDataParams..Option"=w753, "SecondaryDataParams..SecondaryDataVIRef."=w759) -> (w763:T5)
              }
              frame Error {
                n209 = xnode "Error Ring"() -> ("error out"=w765:errorcluster)
              }
            }
          }
          frame "SetSignalBuffer_" {
            n210 = Variant To Data(type=w778, Variant=w780) -> (data=w777:refnum<queue>, error out=w774:errorcluster)  [unwired: 1 in]
            n211 = Select(t=w778, s=w774, f=w777) -> (s? t:f=w779:refnum<queue>)
            n212 = xnode "Error Ring"() -> ("error out"=w773:errorcluster)
            n213 = Select(t=w773, s=w774, f=w775) -> (s? t:f=w776:errorcluster)
          }
          frame "SetMode_" {
            n214 = Unbundle By Name(w797) -> ("Mode"=w794:enum16{"Normal", "Turbo"})
            n215 = Variant To Data(error in=w791, type=w794, Variant=w796) -> (data=w793:enum16{"Normal", "Turbo"}, error out=w792:errorcluster)
            n216 = Select(t=w794, s=w792, f=w793) -> (s? t:f=w795:enum16{"Normal", "Turbo"})
            n217 = Bundle By Name(cluster=w797, "Mode"=w795) -> (w798:T5)
          }
          frame "==AnalogOut==" {
          }
          frame "GetChannelCount_AO" {
            n218 = Unbundle By Name(w815) -> ("Handle_DWF"=w814:i32)
            n219 = call <instrlib>:"Get Channel Count Analog Out.vi"("error in (no error)"=w810, "hdwf"=w814) -> ("error out"=w811:errorcluster, "pcChannel"=w812:i32)  [unwired: 7 in, 1 out]
            n220 = Bundle By Name(cluster=w816, "ChannelCount"=w812) -> (w813:T16)
          }
          frame "fStart_AO" {
            n221 = Unbundle By Name(w831) -> ("Handle_DWF"=w830:i32)
            n222 = Bundle(0, 0) -> (w825:cluster{i32, i32})  [unwired: 1 in]
            n223 = Variant To Data(error in=w822, type=w825, Variant=w829) -> (data=w824:cluster{i32, i32}, error out=w821:errorcluster)
            n224 = case shown="No Error" w821 {
              selector: w821 -> [w836 _]
              tunnel: w830 -> [w841 _]
              tunnel: w824 -> [w840 _]
              tunnel: [w837 w842] -> w823
              frame No Error {
                n225 = Unbundle(w840) -> (w839:i32, w838:i32)
                n226 = call <instrlib>:"fStart Analog Out.vi"("error in (no error)"=w836, "fStart"=w838, "idxChannel"=w839, "hdwf"=w841) -> ("error out"=w837:errorcluster)  [unwired: 6 in, 1 out]
              }
              frame Error {
                n227 = xnode "Error Ring"() -> ("error out"=w842:errorcluster)
              }
            }
          }
          frame "SetChEnable_AO" {
            n228 = Unbundle By Name(w859) -> ("Handle_DWF"=w858:i32)
            n229 = Bundle(0, TRUE) -> (w856:cluster{i32, bool})  [unwired: 1 in]
            n230 = Variant To Data(error in=w853, type=w856, Variant=w857) -> (data=w855:cluster{i32, bool}, error out=w852:errorcluster)
            n231 = case shown="No Error" w852 {
              selector: w852 -> [w871 _]
              tunnel: w858 -> [w872 _]
              tunnel: w855 -> [w868 _]
              tunnel: [w867 w885] -> w854
              tunnel: w851 -> [w870 w884]
              tunnel: [w866 w884] -> w850
              frame No Error {
                n232 = Unbundle(w868) -> (w864:i32, w865:bool)
                n233 = in-place {
                  in-place-border: [w876] -> w869
                  in-place-border: w865 -> [w875]
                  in-place-border: w864 -> [w873]
                  n234 = in-place-cluster #2(w870) -> ("Configs"=w877:T13[])
                  n235 = in-place {
                    in-place-border: [w880] -> w876
                    in-place-border: w875 -> [w879]
                    n236 = in-place-array #3(w877, w873) -> (w881:T13)
                    n237 = in-place {
                      in-place-border: [w882] -> w880
                      in-place-border: w879 -> [w883]
                      n238 = in-place-cluster #4(w881) -> ("Node"=w882:T15)  [unwired: 1 out]
                      n239 = in-place-cluster #4("Enable"=w883, "Node"=w882) -> (w878:T13)
                    }
                    n240 = in-place-array #3(w878) -> (w874:T13[])  [unwired: 1 out]
                  }
                  n241 = in-place-cluster #2("Configs"=w874) -> (w866:T16)
                }
                n242 = call <instrlib>:"Set Channel Enable Analog Out.vi"("fEnable"=w865, "error in (no error)"=w871, "node"=w869, "idxChannel"=w864, "hdwf"=w872) -> ("error out"=w867:errorcluster)  [unwired: 6 in]
              }
              frame Error {
                n243 = xnode "Error Ring"() -> ("error out"=w885:errorcluster)
              }
            }
          }
          frame "SetConfig_AO" {
            n244 = Unbundle By Name(w892) -> ("Configs"=w896:T13[])
            n245 = Unbundle By Name(w903) -> ("Handle_DWF"=w902:i32)
            n246 = Index Array(array=w896) -> (element=w895:T13)  [unwired: 1 in]
            n247 = Bundle(0, w895) -> (w893:cluster{i32, T13})  [unwired: 1 in]
            n248 = Variant To Data(error in=w898, type=w893, Variant=w901) -> (data=w900:cluster{i32, T13}, error out=w897:errorcluster)
            n249 = case shown="No Error" w897 {
              selector: w897 -> [w920 _]
              tunnel: w902 -> [w917 _]
              tunnel: w900 -> [w919 _]
              tunnel: [w916 w946] -> w899
              tunnel: w892 -> [w921 w945]
              tunnel: [w908 w945] -> w891
              frame No Error {
                n250 = Unbundle(w919) -> (w915:i32, w918:T13)
                n251 = Unbundle By Name(w918) -> ("Phase(deg)_AO"=w914:dbl, "Amplitude(V)_AO"=w913:dbl, "Node"=w912:T15, "Frequency(Hz)_AO"=w911:dbl, "Offset(V)_AO"=w910:dbl, "FUNC"=w909:T14)
                n252 = in-place {
                  in-place-border: w915 -> [w929]
                  in-place-border: w914 -> [w928]
                  in-place-border: w913 -> [w927]
                  in-place-border: w912 -> [w926]
                  in-place-border: w911 -> [w925]
                  in-place-border: w910 -> [w924]
                  in-place-border: w909 -> [w923]
                  n253 = in-place-cluster #5(w921) -> ("Configs"=w930:T13[])
                  n254 = in-place {
                    in-place-border: w928 -> [w937]
                    in-place-border: w927 -> [w936]
                    in-place-border: w926 -> [w935]
                    in-place-border: w925 -> [w934]
                    in-place-border: w924 -> [w933]
                    in-place-border: w923 -> [w932]
                    n255 = in-place-array #6(w930, w929) -> (w938:T13)
                    n256 = in-place {
                      in-place-border: w937 -> [w944]
                      in-place-border: w936 -> [w943]
                      in-place-border: w935 -> [w942]
                      in-place-border: w934 -> [w941]
                      in-place-border: w933 -> [w940]
                      in-place-border: w932 -> [w939]
                      n257 = in-place-cluster #7(w938) -> ()  [unwired: 6 out]
                      n258 = in-place-cluster #7("Phase(deg)_AO"=w944, "Amplitude(V)_AO"=w943, "Node"=w942, "Frequency(Hz)_AO"=w941, "Offset(V)_AO"=w940, "FUNC"=w939) -> (w931:T13)
                    }
                    n259 = in-place-array #6(w931) -> (w922:T13[])  [unwired: 1 out]
                  }
                  n260 = in-place-cluster #5("Configs"=w922) -> (w908:T16)
                }
                n261 = call <instrlib>:"Set Config Analog Out.vi"("hdwf"=w917, "vAmplitude"=w913, "degPhase"=w914, "idxChannel"=w915, "node"=w912, "hzFrequency"=w911, "error in (no error)"=w920, "vOffset"=w910, "func"=w909) -> ("error out"=w916:errorcluster)  [unwired: 5 in, 1 out]
              }
              frame Error {
                n262 = xnode "Error Ring"() -> ("error out"=w946:errorcluster)
              }
            }
          }
          frame "SetOffset_AO_" {
            n263 = Unbundle By Name(w953) -> ("Configs"=w957:T13[])
            n264 = Unbundle By Name(w964) -> ("Handle_DWF"=w963:i32)
            n265 = Index Array(array=w957) -> (element=w956:T13)  [unwired: 1 in]
            n266 = Bundle(0, w956) -> (w954:cluster{i32, T13})  [unwired: 1 in]
            n267 = Variant To Data(error in=w959, type=w954, Variant=w962) -> (data=w961:cluster{i32, T13}, error out=w958:errorcluster)
            n268 = case shown="No Error" w958 {
              selector: w958 -> [w970 _]
              tunnel: w963 -> [w975 _]
              tunnel: w961 -> [w977 _]
              tunnel: [w969 w991] -> w960
              tunnel: w953 -> [w978 w990]
              tunnel: [w976 w990] -> w952
              frame No Error {
                n269 = Unbundle(w977) -> (w974:i32, w972:T13)
                n270 = Unbundle By Name(w972) -> ("Offset(V)_AO"=w971:dbl)
                n271 = in-place {
                  in-place-border: w974 -> [w982]
                  in-place-border: [w980] -> w973
                  in-place-border: w971 -> [w979]
                  n272 = in-place-cluster #8(w978) -> ("Configs"=w983:T13[])
                  n273 = in-place {
                    in-place-border: [w985] -> w980
                    in-place-border: w979 -> [w984]
                    n274 = in-place-array #9(w983, w982) -> (w987:T13)
                    n275 = in-place {
                      in-place-border: [w988] -> w985
                      in-place-border: w984 -> [w989]
                      n276 = in-place-cluster #10(w987) -> ("Node"=w988:T15)  [unwired: 1 out]
                      n277 = in-place-cluster #10("Offset(V)_AO"=w989, "Node"=w988) -> (w986:T13)
                    }
                    n278 = in-place-array #9(w986) -> (w981:T13[])  [unwired: 1 out]
                  }
                  n279 = in-place-cluster #8("Configs"=w981) -> (w976:T16)
                }
                n280 = dll-call lib="C:/Windows/System32/dwf.dll" fn="FDwfAnalogOutNodeOffsetSet"(error in=w970, "hdwf"=w975, "idxChannel"=w974, "node"=w973, "vOffset"=w971) -> (error out=w969:errorcluster)  [unwired: 7 in, 1 out]
              }
              frame Error {
                n281 = xnode "Error Ring"() -> ("error out"=w991:errorcluster)
              }
            }
          }
          frame "SetSymetry_AO" {
            n282 = Unbundle By Name(w998) -> ("Configs"=w1002:T13[])
            n283 = Unbundle By Name(w1009) -> ("Handle_DWF"=w1008:i32)
            n284 = Index Array(array=w1002) -> (element=w1001:T13)  [unwired: 1 in]
            n285 = Bundle(0, w1001) -> (w999:cluster{i32, T13})  [unwired: 1 in]
            n286 = Variant To Data(error in=w1004, type=w999, Variant=w1007) -> (data=w1006:cluster{i32, T13}, error out=w1003:errorcluster)
            n287 = case shown="No Error" w1003 {
              selector: w1003 -> [w1022 _]
              tunnel: w1008 -> [w1019 _]
              tunnel: w1006 -> [w1021 _]
              tunnel: [w1018 w1033] -> w1005
              tunnel: w998 -> [w1023 w1032]
              tunnel: [w1015 w1032] -> w997
              frame No Error {
                n288 = Unbundle(w1021) -> (w1017:i32, w1020:T13)
                n289 = Unbundle By Name(w1020) -> ("Symmetry"=w1014:dbl, "Node"=w1016:T15)
                n290 = in-place {
                  in-place-border: w1017 -> [w1026]
                  in-place-border: w1014 -> [w1024]
                  n291 = in-place-cluster #11(w1023) -> ("Configs"=w1027:T13[])
                  n292 = in-place {
                    in-place-border: w1024 -> [w1029]
                    n293 = in-place-array #12(w1027, w1026) -> (w1030:T13)
                    n294 = in-place {
                      in-place-border: w1029 -> [w1031]
                      n295 = in-place-cluster #13(w1030) -> ()  [unwired: 1 out]
                      n296 = in-place-cluster #13("Symmetry"=w1031) -> (w1028:T13)
                    }
                    n297 = in-place-array #12(w1028) -> (w1025:T13[])  [unwired: 1 out]
                  }
                  n298 = in-place-cluster #11("Configs"=w1025) -> (w1015:T16)
                }
                n299 = call <instrlib>:"Set Symmetry Analog Out.vi"("percentageSymmetry"=w1014, "error in (no error)"=w1022, "node"=w1016, "idxChannel"=w1017, "hdwf"=w1019) -> ("error out"=w1018:errorcluster)  [unwired: 5 in, 1 out]
              }
              frame Error {
                n300 = xnode "Error Ring"() -> ("error out"=w1033:errorcluster)
              }
            }
          }
          frame "SetFuncData_AO" {
            n301 = Unbundle By Name(w1040) -> ("Configs"=w1044:T13[])
            n302 = Unbundle By Name(w1051) -> ("Handle_DWF"=w1050:i32)
            n303 = Index Array(array=w1044) -> (element=w1043:T13)  [unwired: 1 in]
            n304 = Bundle(0, w1043) -> (w1041:cluster{i32, T13})  [unwired: 1 in]
            n305 = Variant To Data(error in=w1046, type=w1041, Variant=w1049) -> (data=w1048:cluster{i32, T13}, error out=w1045:errorcluster)
            n306 = case shown="No Error" w1045 {
              selector: w1045 -> [w1065 _]
              tunnel: w1050 -> [w1062 _]
              tunnel: w1048 -> [w1064 _]
              tunnel: [w1061 w1082] -> w1047
              tunnel: w1040 -> [w1066 w1081]
              tunnel: [w1059 w1081] -> w1039
              frame No Error {
                n307 = Unbundle(w1064) -> (w1060:i32, w1063:T13)
                n308 = Unbundle By Name(w1063) -> ("rgdData"=w1057:dbl[], "cData"=w1056:i32)
                n309 = in-place {
                  in-place-border: w1060 -> [w1071]
                  in-place-border: [w1070] -> w1058
                  in-place-border: w1057 -> [w1069]
                  in-place-border: w1056 -> [w1068]
                  n310 = in-place-cluster #14(w1066) -> ("Configs"=w1072:T13[])
                  n311 = in-place {
                    in-place-border: [w1076] -> w1070
                    in-place-border: w1069 -> [w1075]
                    in-place-border: w1068 -> [w1074]
                    n312 = in-place-array #15(w1072, w1071) -> (w1077:T13)
                    n313 = in-place {
                      in-place-border: [w1080] -> w1076
                      in-place-border: w1075 -> [w1079]
                      in-place-border: w1074 -> [w1078]
                      n314 = in-place-cluster #16(w1077) -> ("Node"=w1080:T15)  [unwired: 2 out]
                      n315 = in-place-cluster #16("Node"=w1080, "rgdData"=w1079, "cData"=w1078) -> (w1073:T13)
                    }
                    n316 = in-place-array #15(w1073) -> (w1067:T13[])  [unwired: 1 out]
                  }
                  n317 = in-place-cluster #14("Configs"=w1067) -> (w1059:T16)
                }
                n318 = call <instrlib>:"Set Function Data Analog Out.vi"("cdData"=w1056, "rgdData"=w1057, "error in (no error)"=w1065, "node"=w1058, "idxChannel"=w1060, "hdwf"=w1062) -> ("error out"=w1061:errorcluster)  [unwired: 4 in, 1 out]
              }
              frame Error {
                n319 = xnode "Error Ring"() -> ("error out"=w1082:errorcluster)
              }
            }
          }
          frame "SetStates_AO" {
            n320 = Unbundle By Name(w1091) -> ("States"=w1089:T26)
            n321 = Unbundle By Name(w1100) -> ("Handle_DWF"=w1099:i32)
            n322 = Index Array(array=w1089) -> (element=w1088:T27)  [unwired: 1 in]
            n323 = Bundle(0, "States"=w1088) -> (w1092:T28)  [unwired: 1 in]
            n324 = Variant To Data(error in=w1095, type=w1092, Variant=w1098) -> (data=w1097:T28, error out=w1094:errorcluster)
            n325 = case shown="No Error" w1094 {
              selector: w1094 -> [w1114 _]
              tunnel: w1099 -> [w1113 _]
              tunnel: w1097 -> [w1110 _]
              tunnel: [w1112 w1131] -> w1096
              tunnel: w1091 -> [w1115 w1130]
              tunnel: [w1111 w1130] -> w1090
              frame No Error {
                n326 = Unbundle(w1110) -> (w1108:i32, "States"=w1109:T27)
                n327 = Unbundle By Name(w1109) -> ("Run(s)"=w1105:dbl, "Wait(s)"=w1106:dbl, "cRepeat"=w1107:i32)
                n328 = in-place {
                  in-place-border: w1108 -> [w1120]
                  in-place-border: w1107 -> [w1119]
                  in-place-border: w1106 -> [w1118]
                  in-place-border: w1105 -> [w1117]
                  n329 = in-place-cluster #17(w1115) -> ("States"=w1121:T26)
                  n330 = in-place {
                    in-place-border: w1119 -> [w1125]
                    in-place-border: w1118 -> [w1124]
                    in-place-border: w1117 -> [w1123]
                    n331 = in-place-array #18(w1121, w1120) -> (w1126:T27)
                    n332 = in-place {
                      in-place-border: w1125 -> [w1129]
                      in-place-border: w1124 -> [w1128]
                      in-place-border: w1123 -> [w1127]
                      n333 = in-place-cluster #19(w1126) -> ()  [unwired: 3 out]
                      n334 = in-place-cluster #19("Run(s)"=w1127, "Wait(s)"=w1128, "cRepeat"=w1129) -> (w1122:T27)
                    }
                    n335 = in-place-array #18(w1122) -> (w1116:T26)  [unwired: 1 out]
                  }
                  n336 = in-place-cluster #17("States"=w1116) -> (w1111:T16)
                }
                n337 = call <instrlib>:"Set States Analog Out.vi"("cRepeat"=w1107, "secRun"=w1105, "error in (no error)"=w1114, "secWait"=w1106, "idxChannel"=w1108, "hdwf"=w1113) -> ("error out"=w1112:errorcluster)  [unwired: 4 in, 1 out]
              }
              frame Error {
                n338 = xnode "Error Ring"() -> ("error out"=w1131:errorcluster)
              }
            }
          }
          frame "SetTriggerSource_AO" {
            n339 = Unbundle By Name(w1148) -> ("Handle_DWF"=w1147:i32)
            n340 = Bundle(0, "TriggerSource"=DWF_TrigSrc."None") -> (w1141:cluster{i32, "TriggerSource":T9})  [unwired: 1 in]
            n341 = Variant To Data(error in=w1137, type=w1141, Variant=w1146) -> (data=w1145:cluster{i32, "TriggerSource":T9}, error out=w1143:errorcluster)
            n342 = case shown="No Error" w1143 {
              selector: w1143 -> [w1159 _]
              tunnel: w1147 -> [w1158 _]
              tunnel: w1145 -> [w1155 _]
              tunnel: [w1157 w1170] -> w1144
              tunnel: w1140 -> [w1160 w1169]
              tunnel: [w1156 w1169] -> w1139
              frame No Error {
                n343 = Unbundle(w1155) -> (w1154:i32, "TriggerSource"=w1153:T9)
                n344 = in-place {
                  in-place-border: w1154 -> [w1163]
                  in-place-border: w1153 -> [w1162]
                  n345 = in-place-cluster #20(w1160) -> ("States"=w1164:T26)
                  n346 = in-place {
                    in-place-border: w1162 -> [w1166]
                    n347 = in-place-array #21(w1164, w1163) -> (w1167:T27)
                    n348 = in-place {
                      in-place-border: w1166 -> [w1168]
                      n349 = in-place-cluster #22(w1167) -> ()  [unwired: 1 out]
                      n350 = in-place-cluster #22("TriggerSource"=w1168) -> (w1165:T27)
                    }
                    n351 = in-place-array #21(w1165) -> (w1161:T26)  [unwired: 1 out]
                  }
                  n352 = in-place-cluster #20("States"=w1161) -> (w1156:T16)
                }
                n353 = call <instrlib>:"Set Trigger Source Analog Out.vi"("error in (no error)"=w1159, "trigsrc"=w1153, "idxChannel"=w1154, "hdwf"=w1158) -> ("error out"=w1157:errorcluster)  [unwired: 6 in, 1 out]
              }
              frame Error {
                n354 = xnode "Error Ring"() -> ("error out"=w1170:errorcluster)
              }
            }
          }
          frame "SetMasterNode_AO" {
            # "no implemented yet"
            n355 = Unbundle By Name(w1176) -> ("Configs"=w1181:T13[])
            n356 = Unbundle By Name(w1184) -> ()  [unwired: 1 out]
            n357 = Index Array(array=w1181) -> (element=w1180:T13)  [unwired: 1 in]
            n358 = Bundle(0, w1180) -> (w1178:cluster{i32, T13})  [unwired: 1 in]
            n359 = Variant To Data(error in=w1182, type=w1178, Variant=w1183) -> (error out=w1177:errorcluster)  [unwired: 1 out]
          }
          frame "==Trigger==" {
            n360 = xnode "Error Ring"() -> ("error out"=w1189:errorcluster)
          }
          frame "ManualTrigger" {
            # "add: skip manual trigger if timeout, popup notif. timeout"
            n361 = Unbundle By Name(w1211) -> ("Handle_DWF"=w1208:i32)
            n362 = Tick Count (ms)() -> (millisecond timer value=w1206:u32)
            n363 = for {
              N: 500 -> [_]
              tunnel: w1208 -> [w1221]
              tunnel: [w1220] -> w1207
              tunnel: [w1230] -> w1205
              tunnel: w1206 -> [w1229]
              tunnel: [w1229] -> w1204
              i -> [w1226]
              stop <- w1227 stop-if-true
              w1217 = DWF_DwfState."Done" ("AO1_sts")
              n364 = call <instrlib>:"Get Status Analog In.vi"("hdwf"=w1221) -> ("psts"=w1232:T4, "hdwf out"=w1220:i32)  [unwired: 7 in, 1 out]
              "AI_sts" <- w1232
              n365 = Wait (ms)(milliseconds to wait=u32 1) -> ()  [unwired: 1 out]
              n366 = for {
                N: 2 -> [_]
                tunnel: [w1236] -> w1223 mode=indexing
                tunnel: w1220 -> [w1235]
                i -> [w1234]
                n367 = dll-call lib="C:/Windows/System32/dwf.dll" fn="FDwfAnalogOutStatus"("hdwf"=w1235, "idxChannel"=w1234) -> ("psts"=w1236:i32)  [unwired: 7 in, 2 out]
              }
              n368 = Not Equal?(x=w1232, y=DWF_InstrumentStatus."stsPrefill") -> (x != y?=w1228:bool)
              n369 = Index Array(array=w1223) -> (element #1=w1218:i32, element #2=w1222:i32)  [unwired: 2 in]
              "AO1_sts" <- w1218
              "AO2_sts" <- w1222
              n370 = Less Or Equal?(x=w1218, y=w1217) -> (x <= y?=w1224:bool)
              n371 = Less Or Equal?(x=w1222, y=w1217) -> (x <= y?=w1225:bool)
              n372 = Compound Arithmetic op=AND "AI+AO_Armed"(w1228, w1224, w1225) -> (w1227:bool)
              n373 = Tick Count (ms)() -> (millisecond timer value=w1230:u32)
              "PCTrig_counter" <- w1226
            }
            n374 = Subtract(x=w1205, y=w1204) -> (x-y=→"waited t PCTrig":u32)
            n375 = dll-call lib="C:/Windows/System32/dwf.dll" fn="FDwfDeviceTriggerPC"(error in=w1209, "hdwf"=w1207) -> (error out=w1210:errorcluster)  [unwired: 4 in, 1 out]
            "sysCount_inPCTrig" <- w1201
          }
        }
      }
      frame Error {
        n376 = xnode "Error Ring"() -> ("error out"=w1238:errorcluster)
      }
    }
    n377 = call <userlib>:"ErrorLog.vi"("error in (no error)"=w87) -> ("error out"=w70:errorcluster)  [unwired: 10 in]
  }
  "error out" <- w23
  n378 = while {
    tunnel: w30 -> [w1257]
    tunnel: w32 -> [w1256]
    tunnel: w28 -> [w1254]
    tunnel: w18 -> [w1251]
    tunnel: [w1250] -> w16
    stop <- w1252 stop-if-true
    n379 = event shown="[21] \"SetFuncData_AO\": Value Change" {
      selector: _ -> [_ _ _ _ _ _ _ _ _ _ _ _ _ _ _ _ _ _ _ _ _ _ _]
      dyn-events: _ -> [_ _ _ _ _ _ _ _ _ _ _ _ _ _ _ _ _ _ _ _ _ _ _]
      timeout: 40 -> [_ _ _ _ _ _ _ _ _ _ _ _ _ _ _ _ _ _ _ _ _ _ _]
      tunnel: w1257 -> [w1265 w1269 w1273 w1277 w1281 w1286 w1290 w1297 w1299 w1301 w1303 w1305 w1307 w1309 w1311 w1315 w1317 w1327 w1340 w1346 w1352 w1367 w1375]
      tunnel: w1256 -> [_ _ _ _ _ w1283 _ _ _ _ _ _ _ _ _ _ _ _ _ _ _ _ _]
      tunnel: w1254 -> [w1264 _ _ _ _ _ _ _ _ _ _ _ _ _ _ _ _ _ _ _ _ _ _]
      tunnel: [_ _ _ _ _ _ TRUE _ _ _ _ _ _ _ _ _ _ _ _ _ _ _ _] -> w1253
      tunnel: [w1263 _ _ _ _ _ errorcluster {"status"=FALSE, "code"=0, "source"=""} ("error constant") _ _ _ _ _ _ _ _ _ _ _ _ _ _ _ _] -> w1250
      event Timeout {
        n380 = event-data() -> ()  [unwired: 1 in, 1 out]
        n381 = Bundle By Name(cluster=T1 {"DWF States"=enum."GetStat_", "Variant"=variant} ("element"), "Variant"=w1264) -> (w1261:T1)
        n382 = Enqueue Element At Opposite End "To get LiveStat,\nIt has to be opposite end"(queue=w1265, element=w1261) -> (error out=w1260:errorcluster)  [unwired: 2 in, 2 out]
        n383 = Dequeue Element(queue=w1264, timeout in ms (-1)=100, error in (no error)=w1260) -> (element=→"Live Stats":T5, error out=w1263:errorcluster)  [unwired: 2 out]
      }
      event Value Change {
        n384 = event-data() -> ("NewVal"=w1266:T21)  [unwired: 1 in]
        n385 = Bundle By Name(cluster=T1 {"DWF States"=enum."SetAcquisition_", "Variant"=variant} ("element"), "Variant"=w1266) -> (w1267:T1)
        n386 = Enqueue Element(queue=w1269, element=w1267) -> ()  [unwired: 2 in, 3 out]
      }
      event Value Change {
        n387 = event-data() -> ("NewVal"=w1270:T22)  [unwired: 1 in]
        n388 = Bundle By Name(cluster=T1 {"DWF States"=enum."SetChannels_", "Variant"=variant} ("element"), "Variant"=w1270) -> (w1271:T1)
        n389 = Enqueue Element(queue=w1273, element=w1271) -> ()  [unwired: 2 in, 3 out]
      }
      event Value Change {
        n390 = event-data() -> ("NewVal"=w1274:T23)  [unwired: 1 in]
        n391 = Bundle By Name(cluster=T1 {"DWF States"=enum."SetTrigger_", "Variant"=variant} ("element"), "Variant"=w1274) -> (w1275:T1)
        n392 = Enqueue Element(queue=w1277, element=w1275) -> ()  [unwired: 2 in, 3 out]
      }
      event Value Change {
        n393 = event-data() -> ("NewVal"=w1278:T24)  [unwired: 1 in]
        n394 = Bundle By Name(cluster=T1 {"DWF States"=enum."SetAnalogTrigDetector_", "Variant"=variant} ("element"), "Variant"=w1278) -> (w1279:T1)
        n395 = Enqueue Element(queue=w1281, element=w1279) -> ()  [unwired: 2 in, 3 out]
      }
      event "ConfigAll": Value Change {
        (unwired) T6 {"Acqusition"={"Freq(Hz,SampleRate)"=100000000.0, "BufferSize"=8192, "Mode"=enum."Single", "RecordLength(s)"=0.0}, "Channels"=[{"Range(V)"=5.0, "Offset(V)"=0.0, "Filter"=enum."Decimate", "Enable"=TRUE}], "Trigger"={"TriggerSource"=enum."None", "Timeout(s)"=0.0, "Holdoff(s)"=0.0, "Position/Delay(s)"=0.0}, "AnalogTrigger"={"Channel"=0, "Polarity"=enum."Rising", "Type"=enum."Pulse", "Level(V)"=0.0, "Filter"=enum."Decimate", "Hysterisis(V)"=0.0}} ("Configurations")
        n396 = event-data() -> ()  [unwired: 1 in, 1 out]
        n397 = property class="Clust (strict)"(reference=w1283) -> ("Value"=w1282:T29)  [unwired: 1 in, 2 out]
        n398 = Bundle By Name(cluster=T1 {"DWF States"=enum."SetAll_AcquChTrig_", "Variant"=variant} ("element"), "Variant"=w1282) -> (w1284:T1)
        n399 = Enqueue Element(queue=w1286, element=w1284) -> ()  [unwired: 2 in, 3 out]
      }
      event "Quit": Value Change {
        n400 = event-data() -> ()  [unwired: 1 in, 1 out]
        n401 = Enqueue Element(queue=w1290, element=T1 {"DWF States"=enum."Quit", "Variant"=variant}) -> ()  [unwired: 2 in, 3 out]
      }
      event "Mode(N/T)": Value Change {
        n402 = event-data() -> ("NewVal"=w1291:bool)  [unwired: 1 in]
        n403 = Select(t=enum16{"Normal", "Turbo"}."Turbo" ("Mode"), s=w1291, f=enum16{"Normal", "Turbo"}."Normal" ("Mode")) -> (s? t:f=w1292:enum16{"Normal", "Turbo"})
        n404 = Bundle By Name(cluster=T1 {"DWF States"=enum."SetMode_", "Variant"=variant} ("element"), "Variant"=w1292) -> (w1295:T1)
        n405 = Enqueue Element(queue=w1297, element=w1295) -> ()  [unwired: 2 in, 3 out]
      }
      event "fConfig": Value Change {
        n406 = event-data() -> ()  [unwired: 1 in, 1 out]
        n407 = Enqueue Element(queue=w1299, element=T1 {"DWF States"=enum."fConfigurate", "Variant"=variant}) -> ()  [unwired: 2 in, 3 out]
      }
      event "Start": Value Change {
        n408 = event-data() -> ()  [unwired: 1 in, 1 out]
        n409 = Enqueue Element(queue=w1301, element=T1 {"DWF States"=enum."fStart", "Variant"=variant}) -> ()  [unwired: 2 in, 3 out]
      }
      event "TriggerPC": Value Change {
        n410 = event-data() -> ()  [unwired: 1 in, 1 out]
        n411 = Enqueue Element(queue=w1303, element=T1 {"DWF States"=enum."ManualTrigger", "Variant"=variant}) -> ()  [unwired: 2 in, 3 out]
      }
      event "Reset": Value Change {
        n412 = event-data() -> ()  [unwired: 1 in, 1 out]
        n413 = Enqueue Element(queue=w1305, element=T1 {"DWF States"=enum."Quit", "Variant"=variant}) -> ()  [unwired: 2 in, 3 out]
      }
      event "GetInfo": Value Change {
        n414 = event-data() -> ()  [unwired: 1 in, 1 out]
        n415 = Enqueue Element(queue=w1307, element=T1 {"DWF States"=enum."GetStatus", "Variant"=variant}) -> ()  [unwired: 2 in, 3 out]
      }
      event "CloseAll": Value Change {
        n416 = event-data() -> ()  [unwired: 1 in, 1 out]
        n417 = Enqueue Element(queue=w1309, element=T1 {"DWF States"=enum."CloseAll", "Variant"=variant}) -> ()  [unwired: 2 in, 3 out]
      }
      event "Close": Value Change {
        n418 = event-data() -> ()  [unwired: 1 in, 1 out]
        n419 = Enqueue Element(queue=w1311, element=T1 {"DWF States"=enum."Close", "Variant"=variant}) -> ()  [unwired: 2 in, 3 out]
      }
      event "Open": Value Change {
        n420 = event-data() -> ()  [unwired: 1 in, 1 out]
        n421 = Bundle By Name(cluster=T1 {"DWF States"=enum."Open", "Variant"=variant} ("element"), "Variant"="DevSN") -> (w1313:T1)
        n422 = Enqueue Element(queue=w1315, element=w1313) -> ()  [unwired: 2 in, 3 out]
      }
      event "Enumerate": Value Change {
        n423 = event-data() -> ()  [unwired: 1 in, 1 out]
        n424 = Enqueue Element(queue=w1317, element=T1 {"DWF States"=enum."Enumerate", "Variant"=variant}) -> ()  [unwired: 2 in, 3 out]
      }
      event "SetStates_AO": Value Change {
        n425 = event-data() -> ()  [unwired: 1 in, 1 out]
        n426 = Bundle By Name(cluster=T27 {"Wait(s)"=0.0, "Run(s)"=0.0, "cRepeat"=1, "TriggerSource"=enum."None"} ("States"), "Wait(s)"=0.0, "Run(s)"=0.01, "cRepeat"=1) -> (w1325:T27)
        n427 = Bundle(0, "States"=w1325) -> (w1326:T28)  [unwired: 1 in]
        n428 = Bundle By Name(cluster=T1 {"DWF States"=enum."SetStates_AO", "Variant"=variant} ("element"), "Variant"=w1326) -> (w1319:T1)
        n429 = Enqueue Element(queue=w1327, element=w1319) -> ()  [unwired: 2 in, 3 out]
      }
      event "SetConfig_AO": Value Change {
        w1333 = 100.0  # 1/2 AI sample rate
        w1334 = T14 30 items=["DC"=0, "Sine"=1, "Square"=2, "Triangle"=3, "RampUp"=4, "RampDown"=5, "Noise"=6, "Custom"=30, "Play"=31] ("FUNC")
        n430 = event-data() -> ()  [unwired: 1 in, 1 out]
        n431 = Bundle By Name(cluster=T13 {"FUNC"=3, "Frequency(Hz)_AO"=512.0, "Amplitude(V)_AO"=1.0, "Phase(deg)_AO"=0.0, "Offset(V)_AO"=0.0, "rgdData"=[], "cData"=8192, "Symmetry"=0.0, "Enable"=TRUE, "Node"=enum."Carrier"}, "FUNC"=w1334, "Frequency(Hz)_AO"=w1333, "Amplitude(V)_AO"=1.0, "Phase(deg)_AO"=0.0, "Offset(V)_AO"=0.0, "Enable"=TRUE) -> (w1338:T13)
        n432 = Bundle(0, w1338) -> (w1329:cluster{i32, T13})  [unwired: 1 in]
        n433 = Bundle By Name(cluster=T1 {"DWF States"=enum."SetConfig_AO", "Variant"=variant} ("element"), "Variant"=w1329) -> (w1328:T1)
        n434 = Enqueue Element(queue=w1340, element=w1328) -> ()  [unwired: 2 in, 3 out]
      }
      event "SetEnable_AO": Value Change {
        w1342 = 0  # Channel_1
        n435 = event-data() -> ()  [unwired: 1 in, 1 out]
        n436 = Bundle("Channel_1"=w1342, TRUE) -> (w1343:cluster{"Channel_1":i32, bool})  [unwired: 1 in]
        n437 = Bundle By Name(cluster=T1 {"DWF States"=enum."SetChEnable_AO", "Variant"=variant} ("element"), "Variant"=w1343) -> (w1341:T1)
        n438 = Enqueue Element(queue=w1346, element=w1341) -> ()  [unwired: 2 in, 3 out]
      }
      event "SetTrigSrc_AO": Value Change {
        n439 = event-data() -> ()  [unwired: 1 in, 1 out]
        n440 = Bundle(0, "TriggerSource"=DWF_TrigSrc."PC") -> (w1349:cluster{i32, "TriggerSource":T9})  [unwired: 1 in]
        n441 = Bundle By Name(cluster=T1 {"DWF States"=enum."SetTriggerSource_AO", "Variant"=variant} ("element"), "Variant"=w1349) -> (w1348:T1)
        n442 = Enqueue Element(queue=w1352, element=w1348) -> ()  [unwired: 2 in, 3 out]
      }
      event "SetFuncData_AO": Value Change {
        w1363 = T14 30 items=["DC"=0, "Sine"=1, "Square"=2, "Triangle"=3, "RampUp"=4, "RampDown"=5, "Noise"=6, "Custom"=30, "Play"=31] ("FUNC")
        n443 = event-data() -> ()  [unwired: 1 in, 1 out]
        n444 = disable-structure shown="Disabled" {
          disable-tunnel: 1.0 ("Amplitude") -> [_ _]
          disable-tunnel: 32 ("NumRampPoints") -> [_ _]
          disable-tunnel: 2048 ("NumPoints") -> [_ w1368]
          disable-tunnel: [_ w1369] -> w1357
          frame Disabled {
          }
          frame Enabled {
            n445 = call-poly <vilib>:"Ramp Pattern.vi"("samples"=w1368) -> ("Ramp Pattern"=w1369:dbl[])  [unwired: 9 in, 1 out]
          }
        }
        n446 = Reverse 1D Array(array=w1357) -> (reversed array=w1358:dbl[])
        n447 = Build Array (concatenate)(w1357, w1358) -> (w1359:dbl[])
        n448 = Bundle By Name(cluster=T13 {"FUNC"=3, "Frequency(Hz)_AO"=512.0, "Amplitude(V)_AO"=1.0, "Phase(deg)_AO"=0.0, "Offset(V)_AO"=0.0, "rgdData"=[], "cData"=8192, "Symmetry"=0.0, "Enable"=TRUE, "Node"=enum."Carrier"}, "FUNC"=w1363, "rgdData"=w1359, "cData"=4096) -> (w1365:T13)
        n449 = Bundle(0, w1365) -> (w1355:cluster{i32, T13})  [unwired: 1 in]
        n450 = Bundle By Name(cluster=T1 {"DWF States"=enum."SetFuncData_AO", "Variant"=variant} ("element"), "Variant"=w1355) -> (w1353:T1)
        n451 = Enqueue Element(queue=w1367, element=w1353) -> ()  [unwired: 2 in, 3 out]
      }
      event "fStart_AO": Value Change {
        n452 = event-data() -> ()  [unwired: 1 in, 1 out]
        n453 = Bundle(0, 1) -> (w1372:cluster{i32, i32})  [unwired: 1 in]
        n454 = Bundle By Name(cluster=T1 {"DWF States"=enum."fStart_AO", "Variant"=variant} ("element"), "Variant"=w1372) -> (w1371:T1)
        n455 = Enqueue Element(queue=w1375, element=w1371) -> ()  [unwired: 2 in, 3 out]
      }
    }
    n456 = Or(x=w1253, y=w1251) -> (x .or. y?=w1252:bool)
  }
  n457 = Release Queue(queue=w4) -> ()  [unwired: 2 in, 3 out]
  n458 = Release Queue(queue=w25, error in (no error)=w23) -> (error out=w29:errorcluster)  [unwired: 1 in, 2 out]
  n459 = Release Queue(queue=w30, error in (no error)=w29) -> (error out=w27:errorcluster)  [unwired: 1 in, 2 out]
  n460 = Merge Errors(w16, w27) -> (w17:errorcluster)
  n461 = Release Queue(queue=w28, error in (no error)=w17) -> (error out=w22:errorcluster)  [unwired: 1 in, 2 out]
  n462 = call <vilib>:"General Error Handler.vi"("type of dialog (OK msg:1)"=w21, "error in (no error)"=w22, "[exception action] (none:0)"=w20, "[exception code]"=w19) -> ()  [unwired: 7 in, 5 out]
